vi "simple-LevyLab Analysis Framework (Template).vi"() -> ()   [LabVIEW 2016]
doc: "simple-LevyLab Analysis Framework (s-LLAF).\n\nDrag onto an empty block diagram to make your own."
uses:
  <userlib>/LevyLab/XY Utilities/Typedefs/Interpolation Configuration--cluster.ctl
  <userlib>/LevyLab/Graph Utilities/graph_utilities.lvclass
  <userlib>/LevyLab/Graph Utilities/graph_utilities.lvclass/graph_utilities.ctl
  <userlib>/LevyLab/Graph Utilities/XY Graph/Set XY Graph Value (array).vi
  <userlib>/LevyLab/XY Utilities/subVIs/Add float (multiple).vi
  <userlib>/LevyLab/XY Utilities/subVIs/Subtract float (multiple).vi
  <userlib>/LevyLab/XY Utilities/subVIs/Multiply float (multiple).vi
  <userlib>/LevyLab/XY Utilities/subVIs/Square (multiple).vi
  <userlib>/LevyLab/XY Utilities/subVIs/Divide float (multiple).vi
  <userlib>/LevyLab/XY Utilities/subVIs/Sort (multiple).vi
  <userlib>/LevyLab/XY Utilities/subVIs/Swap X and Y (multiple).vi
  <userlib>/LevyLab/XY Utilities/subVIs/Reverse (multiple).vi
  <userlib>/LevyLab/XY Utilities/subVIs/Subset (multiple).vi
  <userlib>/LevyLab/XY Utilities/subVIs/Derivative (multiple).vi
  <userlib>/LevyLab/XY Utilities/subVIs/Interpolate (multiple).vi
  <userlib>/LevyLab/XY Utilities/subVIs/FFT (multiple).vi
  <userlib>/LevyLab/XY Utilities/subVIs/PS (multiple).vi
  <userlib>/LevyLab/XY Utilities/subVIs/Resample (multiple).vi
  <userlib>/LevyLab/XY Utilities/subVIs/Symmetrize (multiple).vi
  <userlib>/LevyLab/XY Utilities/xy_utilities.lvlib
panel:
  in  "Tab Control":enum32{"Page 1", "Page 2"}(tab)
  in  "STOP":bool
  in  "CLEAR":bool
  out "Current State":string="XY: Load\nGraph: Initialize Graphs\nUI: Display Data"
  in  "Method":enum16{"Slider (%)", "X[] min and max"}(ring)
  in  "Subset Slider":cluster{dbl, dbl}(slide)={0.75, 0.25} caption="Horizontal Slider" scale=0.0..1.0
  in  "Interval":dbl=2.0
  in  "Type":enum16{"dy/dx vs x", "dx/dy vs y"}(ring)
  in  "PROCESS":bool
  in  "Process Queue":string
  in  "Available States":i32(listbox)=-1 caption="States to Process"
  in  "x":dbl format="%#_6p"
  in  "y":dbl format="%#_6p"
  out "Processed States":string="XY: Load\nGraph: Initialize Graphs\nUI: Display Data"
  in  "Interval Units":enum16{"Points", "Data"}(ring)
  in  "Configure":T1={"X Low"=0.05, "X High"=0.5, "X Step"=0.01, "Fake Point"=0.05} {"Fake Point" format="%#_6p"; "X Step" format="%#_6p"; "X High" format="%#_6p"; "X Low" format="%#_6p"}
  in  "Graphs Tab Control":enum32{"Data", "Intensity/Linecuts"}(tab)
  out "XY Graph: Antisymmetric":cluster{"X-array":dbl[], dbl[]}[](graph)
  out "XY Graph: Symmetric":cluster{"X-array":dbl[], dbl[]}[](graph)
  out "XY Graph: Processed":cluster{"Intensity Data":dbl[], "Array":dbl[]}[](graph)
  out "XY Graph: Unprocessed":cluster{"Intensity Data":dbl[], "Array":dbl[]}[](graph)
  out "Data Intensity":dbl[][](graph)
  out "Diff Intensity":dbl[][](graph)
  out "Diff Vertical":cluster{"Array":dbl[], "A x Vector":dbl[]}[](graph)
  out "Diff Horizontal":cluster{"Array":dbl[], "A x Vector":dbl[]}[](graph)
  in  "width (vertical)":dbl=0.2 caption="width"
  in  "width (horizontal)":dbl=0.2 caption="width"
  in  "width (vertical) 2":dbl=0.2 caption="width"
  in  "width (horizontal) 2":dbl=0.2 caption="width"
  out "Data Vertical":cluster{"Array":dbl[], "A x Vector":dbl[]}[](graph)
  out "Data Horizontal":cluster{"Intensity Data":dbl[], "Array":dbl[]}[](graph)
  # "State Scripting"
  # "Process Arguments"
  # "Arithmetic"
  # "Derivative"
  # "Interpolate"
  # "Subset"
  # "\"Process Queue\" is a list of states that will execute when you press the \"PROCESS\" button. (File: Load and Graph: Update Graph are added automatically to the beginning and end of the queue.)\n\nTo add states you can either:\n- Type directly into the Process Queue box.\nor:\n- Select a state in the \"Available States\" box that you want to add to the queue. ctl-v in the \"Process Queue\" control to add to the queue."
  # "XY Graphs"
  # "Symmeterized Graphs"
  # "Data processing (1)"
  # "Data Processing (2)"
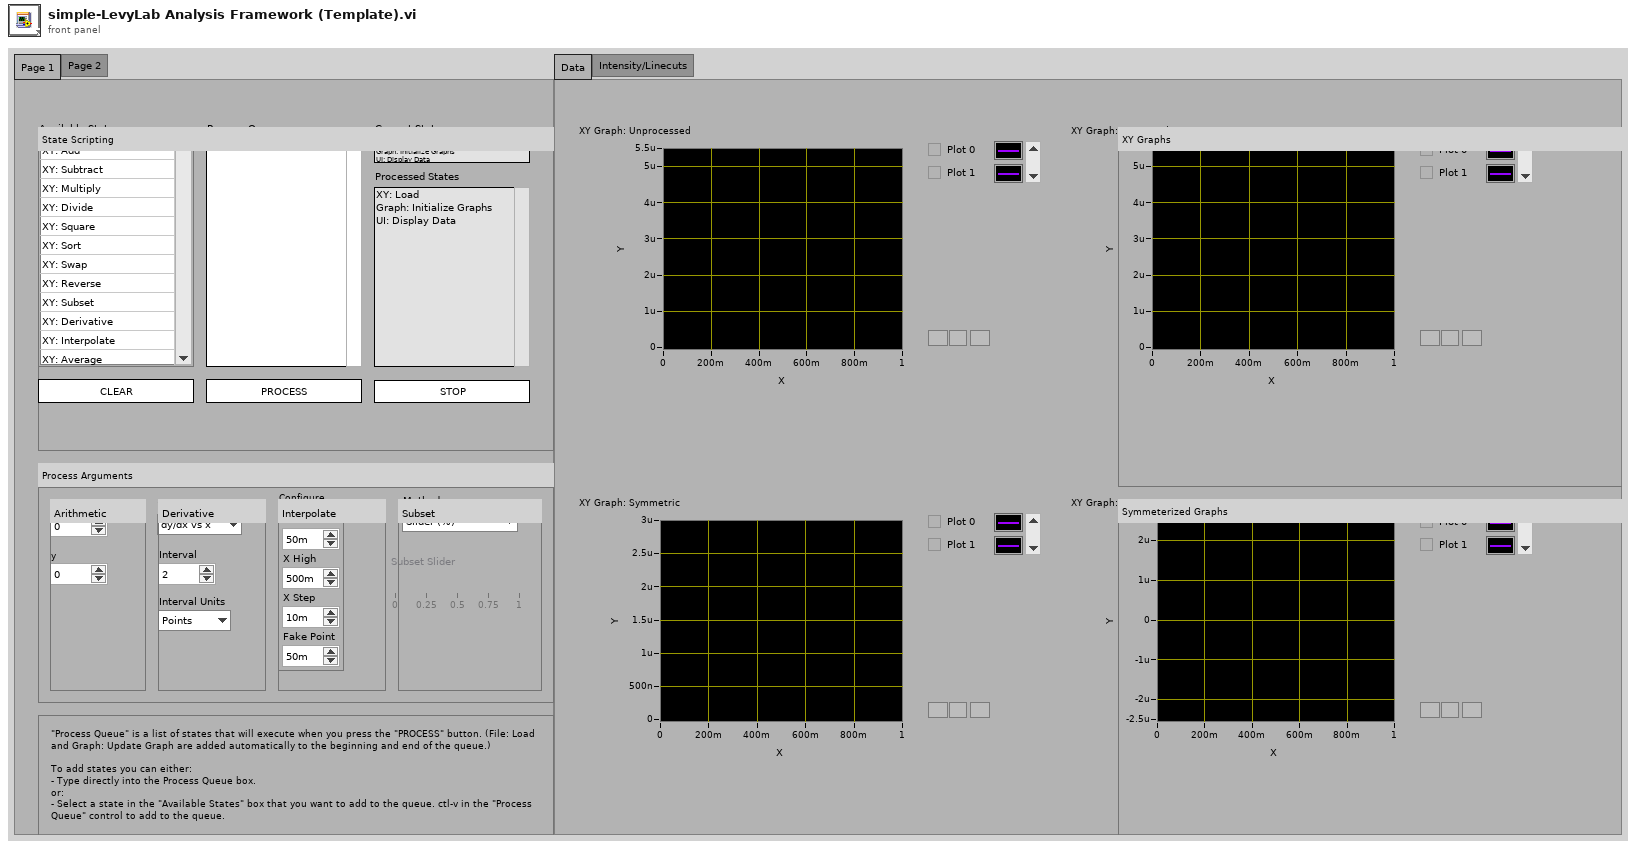
[diagram p1: front panel]
types:
  T1 = typedef "xy_utilities.lvlib/Interpolation Configuration--cluster.ctl" = cluster{"X Low":dbl, "X High":dbl, "X Step":dbl, "Fake Point":dbl}
  T2 = enum32{"Invalid", "Standard", "Closed", "Hidden", "Minimized", "Maximized"}
  T3 = enum32{"invalid app kind", "Development System", "Run Time System", "Student Edition", "Embedded LabVIEW", "Evaluation", "Custom"}
  T4 = cluster{"Shift":bool, "Ctrl":bool, "Alt":bool, "Cmd":bool, "Opt":bool}
  T5 = cluster{"Core":cluster{"Current VI Reference":refnum<vi>, "Close Panel on Exit?":bool}, "Graph":cluster{"Data: Unprocessed":refnum<class "graph_utilities.lvclass">, "Data: Processed":refnum<class "graph_utilities.lvclass">, "Data: Intensity/Vertical":refnum<class "graph_utilities.lvclass">, "Data: Intensity/Horizontal":refnum<class "graph_utilities.lvclass">, "Differential: Intensity/Vertical":refnum<class "graph_utilities.lvclass">, "Differential: Intensity/Horizontal":refnum<class "graph_utilities.lvclass">}, "XY Data (unprocessed)":cluster{"Intensity Data":dbl[], "Array":dbl[]}[], "XY Data (processed 1)":cluster{"Intensity Data":dbl[], "Array":dbl[]}[], "XY Data (processed 2)":cluster{"Intensity Data":dbl[], "Array":dbl[]}[], "Parameter":dbl[]}
  T6 = cluster{"Data: Unprocessed":refnum<class "graph_utilities.lvclass">, "Data: Processed":refnum<class "graph_utilities.lvclass">, "Data: Intensity/Vertical":refnum<class "graph_utilities.lvclass">, "Data: Intensity/Horizontal":refnum<class "graph_utilities.lvclass">, "Differential: Intensity/Vertical":refnum<class "graph_utilities.lvclass">, "Differential: Intensity/Horizontal":refnum<class "graph_utilities.lvclass">}
  T7 = cluster{"Current VI Reference":refnum<vi>, "Close Panel on Exit?":bool}
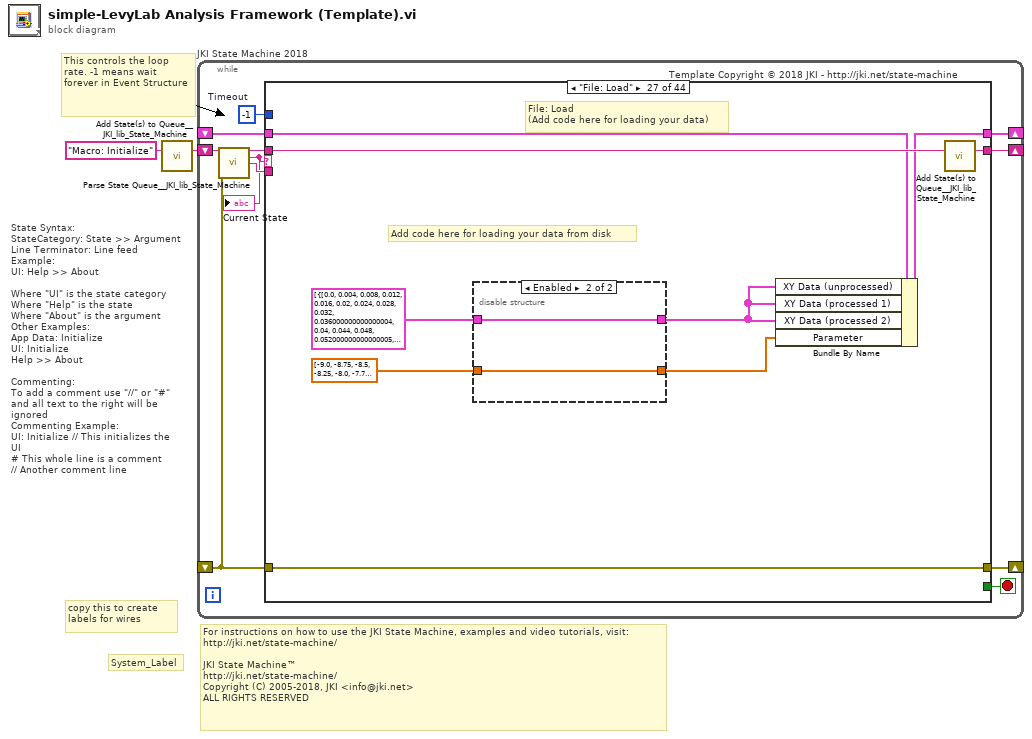
[diagram p0: block diagram]
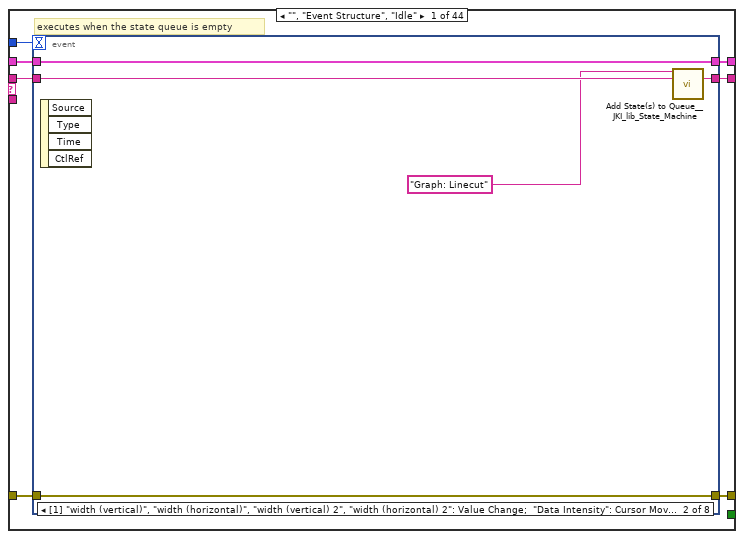
[diagram p2: hidden frame]
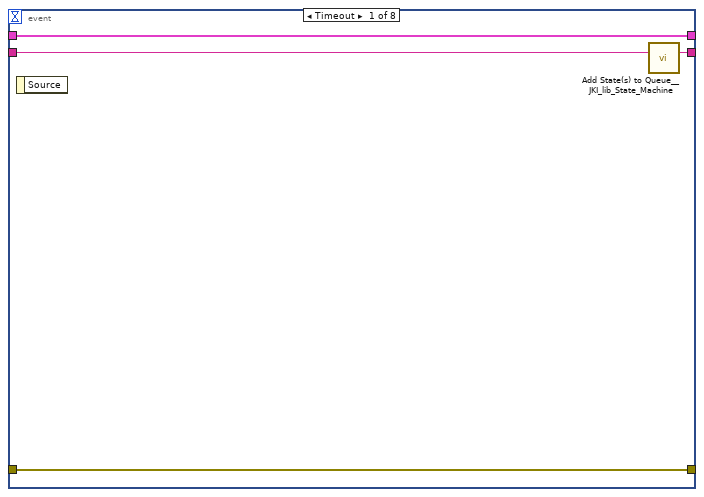
[diagram p3: hidden frame]
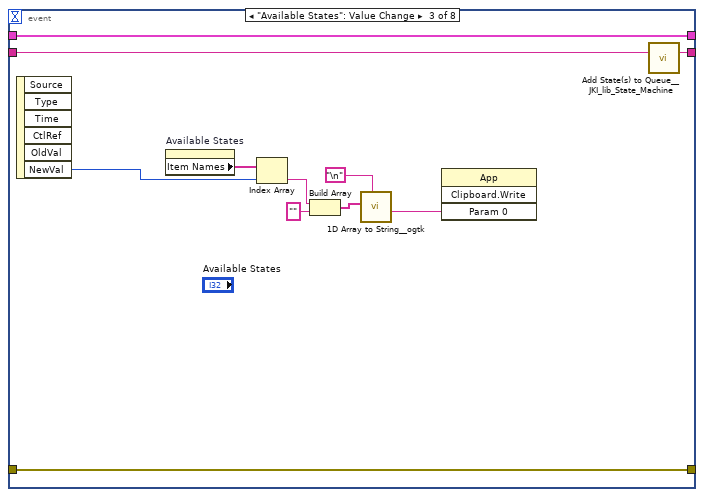
[diagram p4: hidden frame]
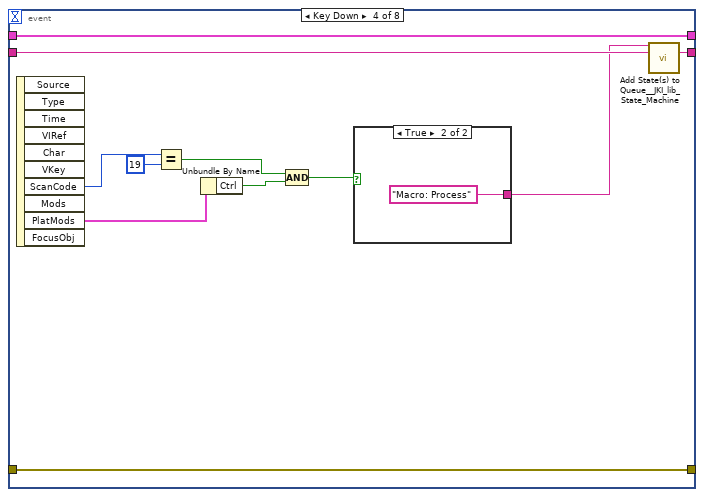
[diagram p5: hidden frame]
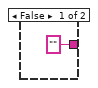
[diagram p6: hidden frame]
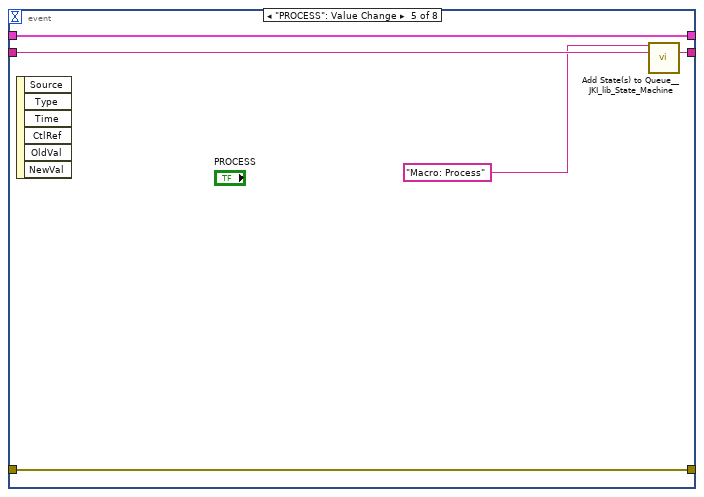
[diagram p7: hidden frame]
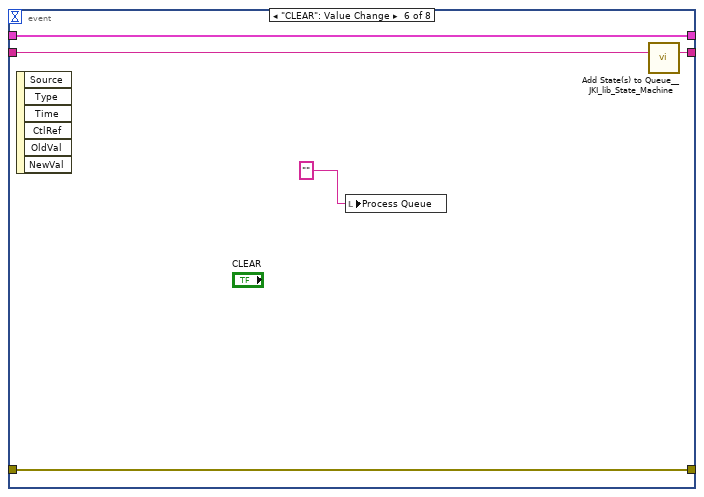
[diagram p8: hidden frame]
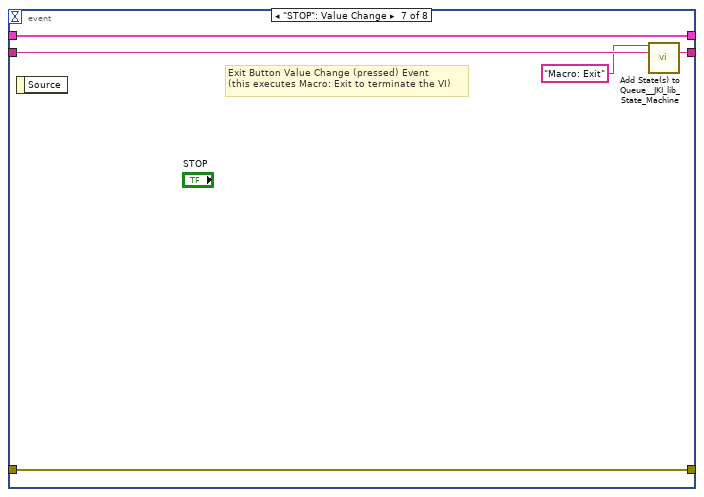
[diagram p9: hidden frame]
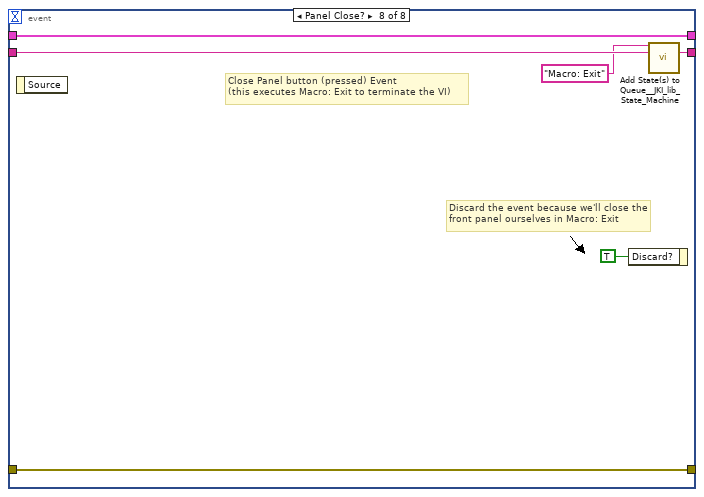
[diagram p10: hidden frame]
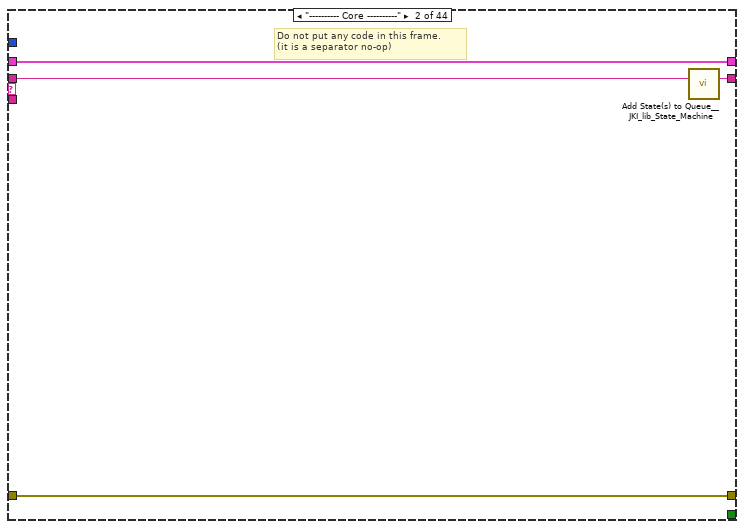
[diagram p11: hidden frame]
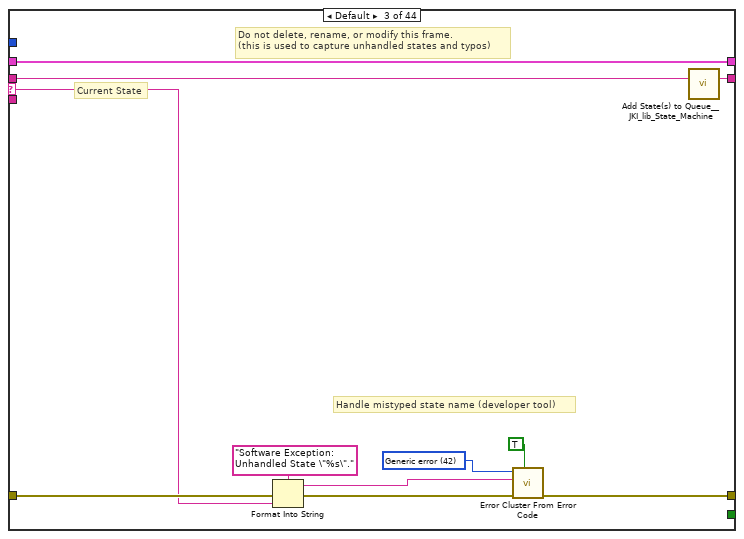
[diagram p12: hidden frame]
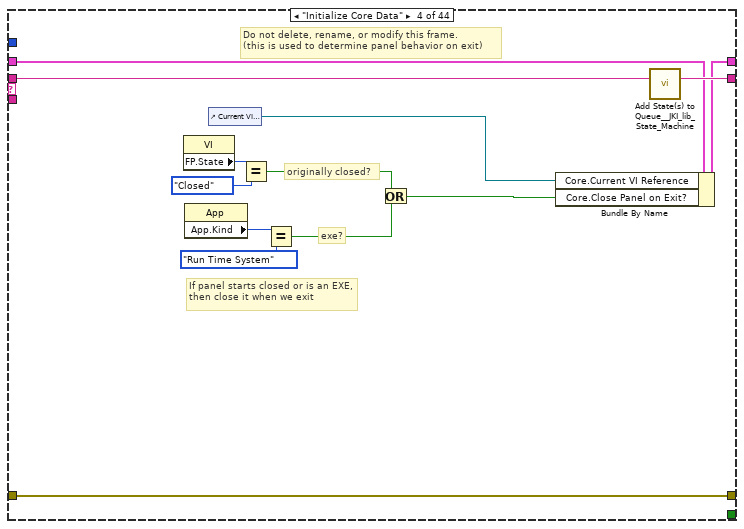
[diagram p13: hidden frame]
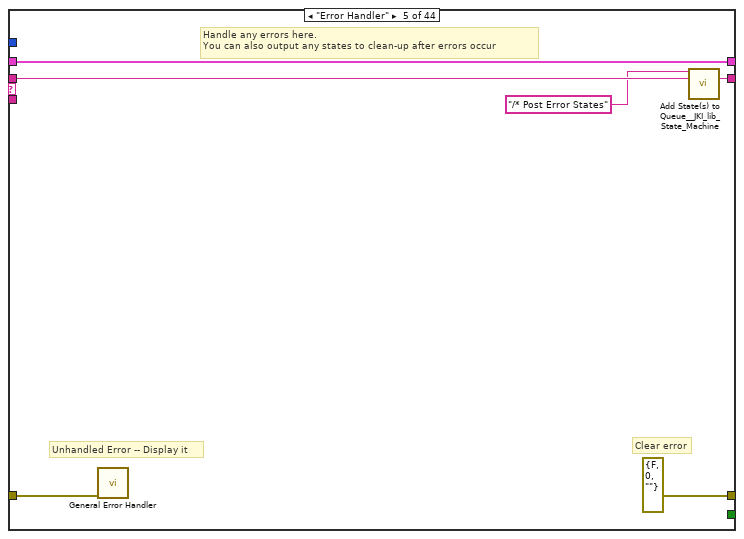
[diagram p14: hidden frame]
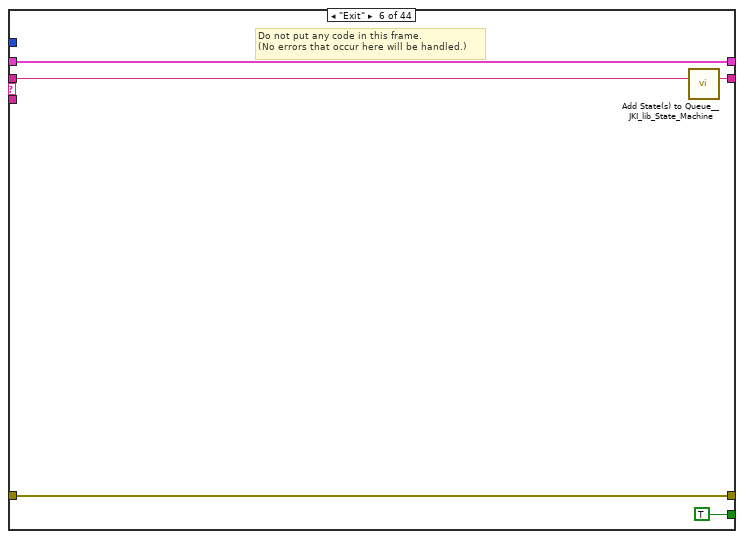
[diagram p15: hidden frame]
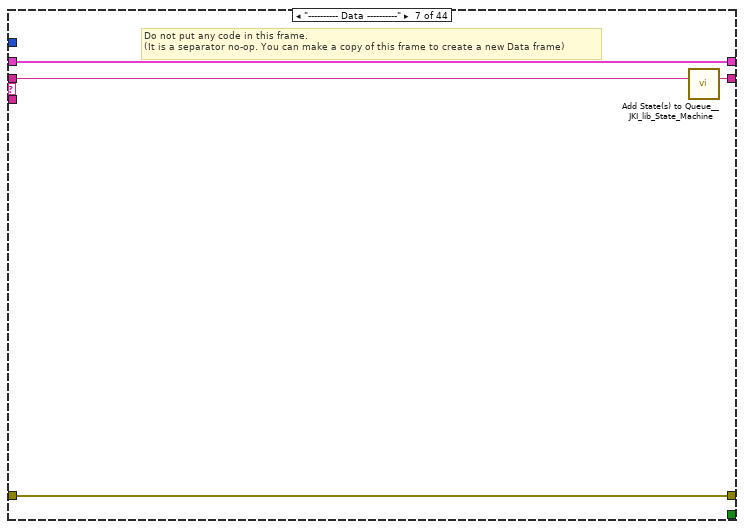
[diagram p16: hidden frame]
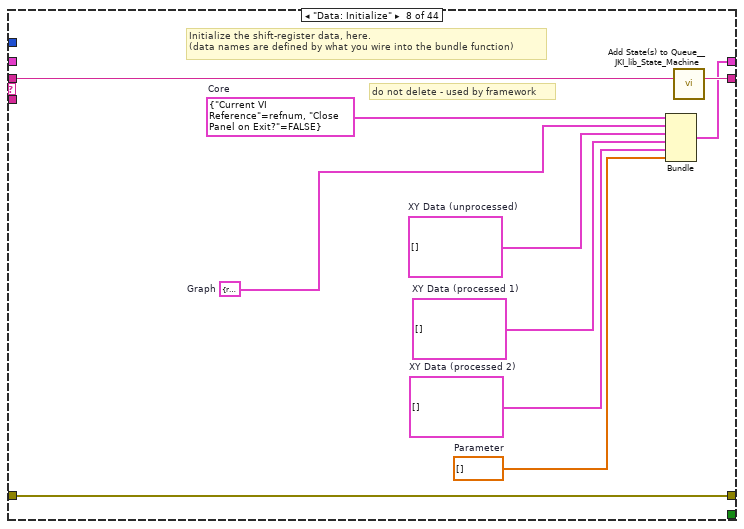
[diagram p17: hidden frame]
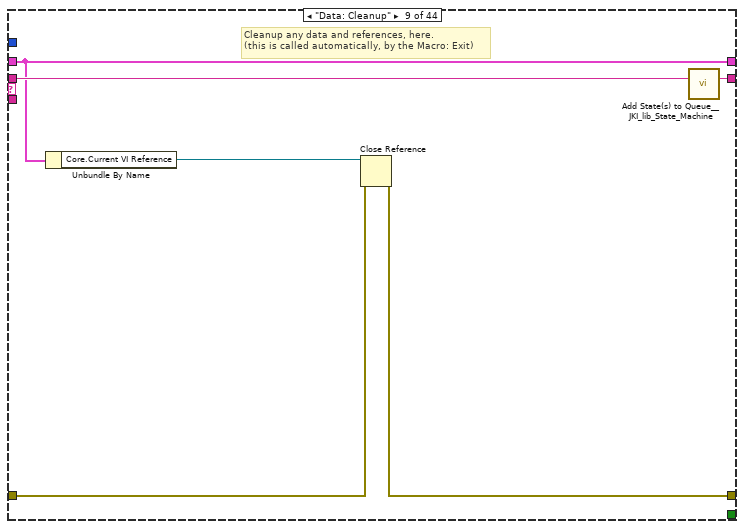
[diagram p18: hidden frame]
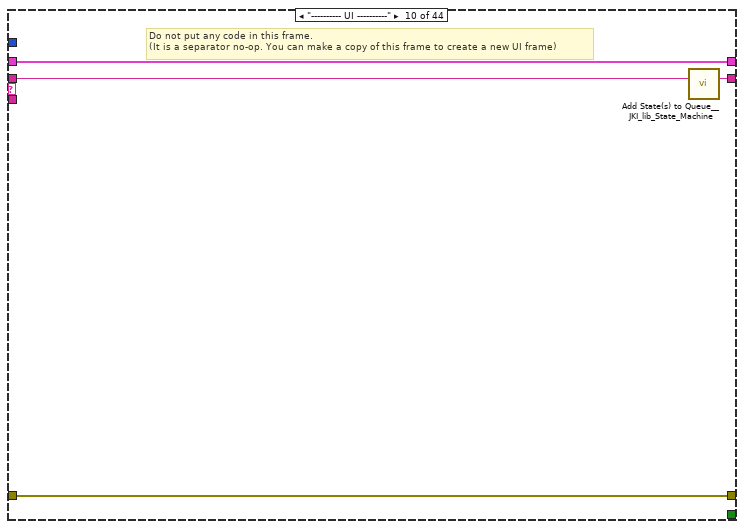
[diagram p19: hidden frame]
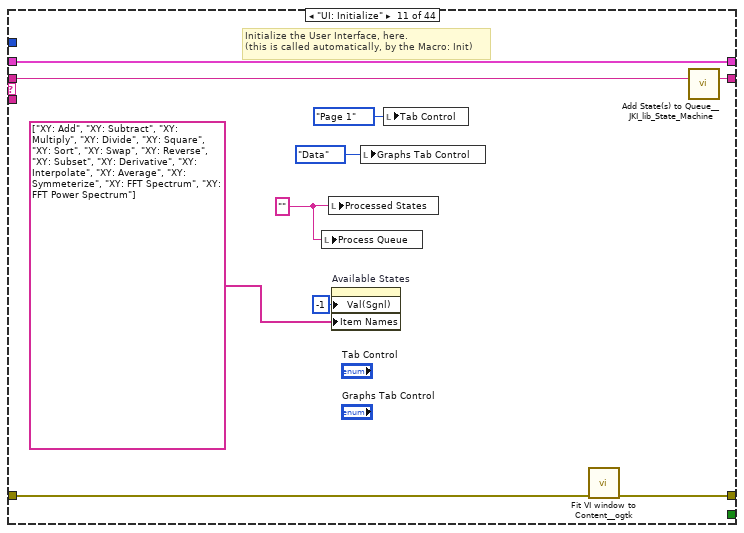
[diagram p20: hidden frame]
diagram:
  # "For instructions on how to use the JKI State Machine, examples and video tutorials, visit:\nhttp://jki.net/state-machine/\n\nJKI State Machine™\nhttp://jki.net/state-machine/\nCopyright (C) 2005-2018, JKI <info@jki.net>\nALL RIGHTS RESERVED"
  # "State Syntax:\nStateCategory: State >> Argument\nLine Terminator: Line feed\nExample:\nUI: Help >> About\n\nWhere \"UI\" is the state category\nWhere \"Help\" is the state\nWhere \"About\" is the argument\nOther Examples:\nApp Data: Initialize\nUI: Initialize\nHelp >> About\n\nCommenting:\nTo add a comment use \"//\" or \"#\" and all text to the right will be ignored\nCommenting Example:\nUI: Initialize // This initializes the UI\n# This whole line is a comment\n// Another comment line"
  # "copy this to create labels for wires"
  # "This controls the loop rate. -1 means wait forever in Event Structure"
  # "System_Label"
  n1 = call <vilib>:"Add State(s) to Queue__JKI_lib_State_Machine.vi"("State(s) in (\"\")"="Macro: Initialize") -> ("States Out"=w2:string)  [unwired: 14 in]
  n2 = while "JKI State Machine 2018" {
    shift-right: [w7] -> _
    shift-left: _ -> [w6]
    shift-right: [w10] -> _
    shift-left: _ -> [w4]
    shift-right: [w9] -> _
    shift-left: w2 -> [w11]
    stop <- w8 stop-if-true
    w5 = -1  # Timeout
    # "Template Copyright © 2018 JKI - http://jki.net/state-machine"
    n3 = call <vilib>:"Parse State Queue__JKI_lib_State_Machine.vi"("State Queue"=w11, "Error In (no error)"=w4) -> ("Remaining States"=w13:string, "Current State"=w3:string, "Arguments"=w12:string)  [unwired: 11 in]
    "Current State" <- w3
    n4 = case shown="\"File: Load\"" w3 {
      selector: w3 -> [_ _ w79 _ _ _ _ _ _ _ _ _ _ _ _ _ _ _ _ _ _ _ _ _ _ _ _ _ _ _ _ _ _ _ _ _ _ _ _ _ _ _ _ _]
      tunnel: w13 -> [w20 w78 w83 w102 w108 w113 w117 w127 w133 w137 w147 w153 w164 w233 w238 w248 w256 w260 w264 w281 w305 w315 w325 w349 w365 w369 w378 w392 w402 w412 w422 w430 w440 w448 w456 w464 w474 w485 w494 w502 w510 w518 w526 w536]
      tunnel: w12 -> [_ _ _ _ _ _ _ _ _ _ _ w148 w158 _ _ _ _ _ _ _ _ _ _ _ _ _ _ _ _ _ _ _ _ _ _ _ _ _ _ _ _ _ _ _]
      tunnel: w6 -> [w18 w75 w81 w95 w105 w111 w114 _ w128 w134 w145 w151 w160 w230 w235 w245 w253 w257 w261 w279 w303 w310 w323 w346 w363 w366 w373 w389 w399 w409 w419 w427 w437 w445 w453 w461 w471 w482 w491 w499 w507 w515 w523 w533]
      tunnel: [w17 w76 w85 w99 errorcluster {"status"=FALSE, "code"=0, "source"=""} ("error out") w110 w115 w124 w129 w135 w138 w149 w161 w231 w236 w246 w254 w258 w262 w277 w288 w306 w316 w347 w354 w367 w370 w385 w395 w405 w415 w423 w433 w441 w449 w457 w467 w479 w487 w495 w504 w511 w519 w529] -> w10
      tunnel: w4 -> [w16 w76 w84 w99 w104 w110 w115 w124 w130 w135 w139 w150 w162 w231 w236 w246 w254 w258 w262 w268 w282 w309 w320 w347 w356 w367 w370 w386 w396 w406 w416 w424 w434 w442 w450 w458 w468 w480 w488 w496 w505 w512 w520 w530]
      tunnel: [w19 w77 w82 w101 w107 w112 w116 w126 w132 w136 w146 w152 w163 w232 w237 w247 w255 w259 w263 w280 w304 w314 w324 w348 w364 w368 w377 w391 w401 w411 w421 w429 w439 w447 w455 w463 w473 w484 w493 w501 w509 w517 w525 w535] -> w9
      tunnel: [_ _ _ _ _ TRUE _ _ _ _ _ _ _ _ _ _ _ _ _ _ _ _ _ _ _ _ _ _ _ _ _ _ _ _ _ _ _ _ _ _ _ _ _ _] -> w8
      tunnel: [w15 w75 w81 w100 w105 w111 w114 w125 w128 w134 w145 w151 w160 w230 w235 w245 w253 w257 w261 w278 w302 w310 w323 w346 w363 w366 w376 w388 w398 w408 w418 w426 w436 w444 w452 w460 w470 w481 w490 w498 w506 w514 w522 w532] -> w7
      tunnel: w5 -> [w14 _ _ _ _ _ _ _ _ _ _ _ _ _ _ _ _ _ _ _ _ _ _ _ _ _ _ _ _ _ _ _ _ _ _ _ _ _ _ _ _ _ _ _]
      frame "", "Event Structure", "Idle" {
        # "executes when the state queue is empty"
        n5 = event shown="[1] \"width (vertical)\", \"width (horizontal)\", \"width (vertical) 2\", \"width (horizontal) 2\": Value Change;  \"Data Intensity\": Cursor Move" {
          selector: _ -> [_ _ _ _ _ _ _ _]
          dyn-events: _ -> [_ _ _ _ _ _ _ _]
          timeout: w14 -> [_ _ _ _ _ _ _ _]
          tunnel: w20 -> [w24 w29 w40 w51 w58 w63 w68 w74]
          tunnel: [w23 w28 w39 w50 w57 w62 w67 w73] -> w19
          tunnel: w18 -> [w21 w26 w37 w48 w55 w60 w65 w71]
          tunnel: [w22 w27 w38 w49 w56 w61 w66 w72] -> w17
          tunnel: w16 -> [w22 w27 w38 w49 w56 w61 w66 w72]
          tunnel: [w21 w26 w37 w48 w55 w60 w65 w71] -> w15
          event Timeout {
            n6 = event-data() -> ()  [unwired: 1 in, 1 out]
            n7 = call <vilib>:"Add State(s) to Queue__JKI_lib_State_Machine.vi"("State(s) in (\"\")"=w24) -> ("States Out"=w23:string)  [unwired: 14 in]
          }
          event "width (vertical)", "width (horizontal)", "width (vertical) 2", "width (horizontal) 2": Value Change; "Data Intensity": Cursor Move {
            n8 = event-data() -> ()  [unwired: 1 in, 4 out]
            n9 = call <vilib>:"Add State(s) to Queue__JKI_lib_State_Machine.vi"("State(s) in Front (\"\")"="Graph: Linecut" ("State(s) in Front (\"\")"), "State(s) in (\"\")"=w29) -> ("States Out"=w28:string)  [unwired: 13 in]
          }
          event "Available States": Value Change {
            n10 = event-data() -> ("NewVal"=w31:i32)  [unwired: 1 in, 5 out]
            n11 = property on="Available States" class="LstBox (strict)"() -> ("Item Names"=w32:string[])  [unwired: 2 in, 2 out]
            n12 = Index Array(array=w32, index=w31) -> (element=w36:string)
            n13 = Build Array(w36, "" ("element")) -> (w33:string[])
            n14 = call <userlib>:"1D Array to String__ogtk.vi"("delimiter (Tab)"="\n", "Array of Strings"=w33) -> ("delimited string"=w34:string)  [unwired: 9 in]
            n15 = invoke class="App" method="Clipboard.Write"("Param 0"=w34) -> ()  [unwired: 3 in, 4 out]
            n16 = call <vilib>:"Add State(s) to Queue__JKI_lib_State_Machine.vi"("State(s) in (\"\")"=w40) -> ("States Out"=w39:string)  [unwired: 14 in]
          }
          event Key Down {
            n17 = event-data() -> ("ScanCode"=w41:i16, "PlatMods"=w42:T4)  [unwired: 1 in, 8 out]
            n18 = Equal?(x=w41, y=i16 19) -> (x = y?=w44:bool)
            n19 = Unbundle By Name(w42) -> ("Ctrl"=w45:bool)
            n20 = Compound Arithmetic op=AND(w44, w45) -> (w43:bool)
            n21 = case shown="True" w43 {
              tunnel: ["" ("State(s) in Front (\"\")") "Macro: Process" ("State(s) in Front (\"\")")] -> w46
              frame False {
              }
              frame True {
              }
            }
            n22 = call <vilib>:"Add State(s) to Queue__JKI_lib_State_Machine.vi"("State(s) in Front (\"\")"=w46, "State(s) in (\"\")"=w51) -> ("States Out"=w50:string)  [unwired: 13 in]
          }
          event "PROCESS": Value Change {
            n23 = event-data() -> ()  [unwired: 1 in, 6 out]
            n24 = call <vilib>:"Add State(s) to Queue__JKI_lib_State_Machine.vi"("State(s) in Front (\"\")"="Macro: Process" ("State(s) in Front (\"\")"), "State(s) in (\"\")"=w58) -> ("States Out"=w57:string)  [unwired: 13 in]
          }
          event "CLEAR": Value Change {
            n25 = event-data() -> ()  [unwired: 1 in, 6 out]
            n26 = local write "Process Queue"("" ("Process States")) -> ()
            n27 = call <vilib>:"Add State(s) to Queue__JKI_lib_State_Machine.vi"("State(s) in (\"\")"=w63) -> ("States Out"=w62:string)  [unwired: 14 in]
          }
          event "STOP": Value Change {
            # "Exit Button Value Change (pressed) Event\n(this executes Macro: Exit to terminate the VI)"
            n28 = event-data() -> ()  [unwired: 1 in, 1 out]
            n29 = call <vilib>:"Add State(s) to Queue__JKI_lib_State_Machine.vi"("State(s) in Front (\"\")"="Macro: Exit", "State(s) in (\"\")"=w68) -> ("States Out"=w67:string)  [unwired: 13 in]
          }
          event Panel Close? {
            # "Discard the event because we'll close the front panel ourselves in Macro: Exit"
            # "Close Panel button (pressed) Event\n(this executes Macro: Exit to terminate the VI)"
            n30 = event-data() -> ()  [unwired: 1 in, 1 out]
            n31 = event-data("Discard?"=TRUE) -> ()  [unwired: 1 in, 1 out]
            n32 = call <vilib>:"Add State(s) to Queue__JKI_lib_State_Machine.vi"("State(s) in Front (\"\")"="Macro: Exit", "State(s) in (\"\")"=w74) -> ("States Out"=w73:string)  [unwired: 13 in]
          }
        }
      }
      frame "---------- Core ----------" {
        # "Do not put any code in this frame.\n(it is a separator no-op)"
        n33 = call <vilib>:"Add State(s) to Queue__JKI_lib_State_Machine.vi"("State(s) in (\"\")"=w78) -> ("States Out"=w77:string)  [unwired: 14 in]
      }
      frame Default {
        w88 = 42 items=["No error", "Argument error", "Memory is full", "Out of zone", "End of file", "File already open", "Generic file I/O error", "File not found", "File permission error", "Disk is full", "Duplicate path", "Too many files open", "System feature not enabled", "Resource file not found", "Cannot add resource", "Resource not found", "Image not found", "Image memory error", "Pen does not exist", "Config type invalid", "Config token not found", "Config parse error", "Config memory error", "Bad external code format", "Bad external code offset", "External code not present", "Null window", "Destroy window error", "Null menu", "Print aborted", "Bad print record", "Print driver error", "Windows error during printing", "Memory error during printing", "Print dialog error", "Generic print error", "Invalid device refnum", "Device not found", "Device parameter error", "Device unit error", "Cannot open device", "Device call aborted", "Generic error", "Cancelled by user", "Object ID too low", "Object ID too high", "Object not in heap", "Unknown heap", "Unknown object (invalid DefProc)", "Unknown object (DefProc not in table)", "Message out of range", "Invalid (null) method", "Unknown message", "Manager call not supported", "Bad address", "Network operation in progress", "Network operation timed out", "Connection is busy", "Network attribute not supported", "Network error", "Address in use", "System out of memory", "Connection aborted", "Connection refused", "Not connected", "Already connected", "Connection closed", "Initialization error (interapplication manager)", "Bad occurrence", "Wait on unbound occurrence handler", "Occurrence queue overflow", "Datalog type conflict", "Unused", "Unrecognized type (interapplication manager)", "Memory corrupt", "Failed to make temporary DLL", "Old CIN version", "Drag socket not found", "Failed to load drop-object", "Failed to register OLE object", "Failed to release OLE object", "Format specifier type mismatch", "Unknown format specifier", "Too few format specifiers", "Too many format specifiers", "Scan failed", "Newer CIN version", "Error converting to variant", "Runtime menu error", "Password tampered", "Variant attribute not found", "Incompatible variant data type", "Event data is not available", "Event Store is not present", "Occurrence is not found", "Event Queue is not created", "Event info is not available", "Refnum passed is NULL", "Error retrieving Class GUID", "Error retrieving CoClass GUID", "Error retrieving TypeLib GUID.", "Bad built application magic bytes.", "Specific driver is different from the specific driver associated with the Logical Name.", "There is no session opened to the class driver.", "Max Error", "MAX - Error with config objects", "MAX - Error loading configuration", "MAX - Group not supported"]
        # "Current State"
        # "Do not delete, rename, or modify this frame.\n(this is used to capture unhandled states and typos)"
        # "Handle mistyped state name (developer tool)"
        n34 = Format Into String(format string="Software Exception: Unhandled State \"%s\"." ("message"), error in=w84, w79) -> (resulting string=w87:string, error out=w86:errorcluster)  [unwired: 1 in]
        n35 = call <vilib>:"Error Cluster From Error Code.vi"("show call chain? (False)"=TRUE, "error in (no error)"=w86, "error message (\"\")"=w87, "error code (0)"=w88) -> ("error out"=w85:errorcluster)  [unwired: 5 in]
        n36 = call <vilib>:"Add State(s) to Queue__JKI_lib_State_Machine.vi"("State(s) in (\"\")"=w83) -> ("States Out"=w82:string)  [unwired: 14 in]
      }
      frame "Initialize Core Data" {
        # "Do not delete, rename, or modify this frame.\n(this is used to determine panel behavior on exit)"
        # "originally closed?"
        # "exe?"
        # "If panel starts closed or is an EXE, then close it when we exit"
        n37 = property class="VI"() -> ("FP.State"=w92:T2)  [unwired: 2 in, 2 out]
        n38 = property class="App"() -> ("App.Kind"=w98:T3)  [unwired: 2 in, 2 out]
        n39 = control-ref of="Current VI Reference"() -> (w93:refnum<vi>)
        n40 = Equal?(x=w92, y=T2."Closed" ("Front Panel Window:State")) -> (x = y?=w90:bool)
        n41 = Equal?(x=w98, y=T3."Run Time System" ("Application:Kind")) -> (x = y?=w96:bool)
        n42 = Or(x=w90, y=w96) -> (x .or. y?=w94:bool)
        n43 = Bundle By Name(cluster=w95, "Core.Current VI Reference"=w93, "Core.Close Panel on Exit?"=w94) -> (w100:T5)
        n44 = call <vilib>:"Add State(s) to Queue__JKI_lib_State_Machine.vi"("State(s) in (\"\")"=w102) -> ("States Out"=w101:string)  [unwired: 14 in]
      }
      frame "Error Handler" {
        # "Unhandled Error -- Display it"
        # "Handle any errors here.\nYou can also output any states to clean-up after errors occur"
        # "Clear error"
        n45 = call <vilib>:"General Error Handler.vi"("error in (no error)"=w104) -> ()  [unwired: 10 in, 5 out]
        n46 = call <vilib>:"Add State(s) to Queue__JKI_lib_State_Machine.vi"("State(s) in Front (\"\")"="/* Post Error States", "State(s) in (\"\")"=w108) -> ("States Out"=w107:string)  [unwired: 13 in]
      }
      frame "Exit" {
        # "Do not put any code in this frame.\n(No errors that occur here will be handled.)"
        n47 = call <vilib>:"Add State(s) to Queue__JKI_lib_State_Machine.vi"("State(s) in (\"\")"=w113) -> ("States Out"=w112:string)  [unwired: 14 in]
      }
      frame "---------- Data ----------" {
        # "Do not put any code in this frame.\n(It is a separator no-op. You can make a copy of this frame to create a new Data frame)"
        n48 = call <vilib>:"Add State(s) to Queue__JKI_lib_State_Machine.vi"("State(s) in (\"\")"=w117) -> ("States Out"=w116:string)  [unwired: 14 in]
      }
      frame "Data: Initialize" {
        w118 = T6 {"Data: Unprocessed"=refnum, "Data: Processed"=refnum, "Data: Intensity/Vertical"=refnum, "Data: Intensity/Horizontal"=refnum, "Differential: Intensity/Vertical"=refnum, "Differential: Intensity/Horizontal"=refnum}  # Graph
        w119 = cluster{"Intensity Data":dbl[], "Array":dbl[]}[] []  # XY Data (processed 2)
        w120 = dbl[] []  # Parameter
        w121 = cluster{"Intensity Data":dbl[], "Array":dbl[]}[] []  # XY Data (processed 1)
        w122 = cluster{"Intensity Data":dbl[], "Array":dbl[]}[] []  # XY Data (unprocessed)
        w123 = T7 {"Current VI Reference"=refnum, "Close Panel on Exit?"=FALSE}  # Core
        # "do not delete - used by framework"
        # "Initialize the shift-register data, here.\n(data names are defined by what you wire into the bundle function)"
        n49 = Bundle("Core"=w123, "Graph"=w118, "XY Data (unprocessed)"=w122, "XY Data (processed 1)"=w121, "XY Data (processed 2)"=w119, "Parameter"=w120) -> (w125:T5)  [unwired: 1 in]
        n50 = call <vilib>:"Add State(s) to Queue__JKI_lib_State_Machine.vi"("State(s) in (\"\")"=w127) -> ("States Out"=w126:string)  [unwired: 14 in]
      }
      frame "Data: Cleanup" {
        # "Cleanup any data and references, here.\n(this is called automatically, by the Macro: Exit)"
        n51 = Unbundle By Name(w128) -> ("Core.Current VI Reference"=w131:refnum<vi>)
        n52 = Close Reference(reference=w131, error in (no error)=w130) -> (error out=w129:errorcluster)
        n53 = call <vilib>:"Add State(s) to Queue__JKI_lib_State_Machine.vi"("State(s) in (\"\")"=w133) -> ("States Out"=w132:string)  [unwired: 14 in]
      }
      frame "---------- UI ----------" {
        # "Do not put any code in this frame.\n(It is a separator no-op. You can make a copy of this frame to create a new UI frame)"
        n54 = call <vilib>:"Add State(s) to Queue__JKI_lib_State_Machine.vi"("State(s) in (\"\")"=w137) -> ("States Out"=w136:string)  [unwired: 14 in]
      }
      frame "UI: Initialize" {
        w141 = "" ("Process States")
        # "Initialize the User Interface, here.\n(this is called automatically, by the Macro: Init)"
        n55 = local write "Process Queue"(w141) -> ()
        n56 = local write "Processed States"(w141) -> ()
        n57 = property on="Available States" class="LstBox (strict)"("Val(Sgnl)"=-1 ("Value (Signaling)"), "Item Names"=string[] ["XY: Add", "XY: Subtract", "XY: Multiply", "XY: Divide", "XY: Square", "XY: Sort", "XY: Swap", "XY: Reverse", "XY: Subset", "XY: Derivative", "XY: Interpolate", "XY: Average", "XY: Symmeterize", "XY: FFT Spectrum", "XY: FFT Power Spectrum"]) -> ()  [unwired: 2 in, 2 out]
        n58 = local write "Graphs Tab Control"(enum32{"Data", "Intensity/Linecuts"}."Data" ("Graphs Tab Control")) -> ()
        n59 = local write "Tab Control"(enum32{"Page 1", "Page 2"}."Page 1" ("Tab Control")) -> ()
        n60 = call <userlib>:"Fit VI window to Content__ogtk.vi"("error in (no error)"=w139) -> ("error out"=w138:errorcluster)  [unwired: 5 in, 1 out]
        n61 = call <vilib>:"Add State(s) to Queue__JKI_lib_State_Machine.vi"("State(s) in (\"\")"=w147) -> ("States Out"=w146:string)  [unwired: 14 in]
      }
      frame "UI: Cursor Set" {
        # "Argument"
        # "Set and Unset Cursor Busy.\n(Usage: \"UI: Cursor Set >> Busy|Idle\")"
        n62 = case shown="\"Idle\", Default" w148 {
          tunnel: w150 -> [w155 w157]
          tunnel: [w154 w156] -> w149
          frame "Idle", Default {
            n63 = call <vilib>:"Unset Busy.vi"("error in (no error)"=w155) -> ("error out"=w154:errorcluster)  [unwired: 10 in]
          }
          frame "Busy" {
            n64 = call <vilib>:"Set Busy.vi"("error in (no error)"=w157) -> ("error out"=w156:errorcluster)  [unwired: 9 in, 1 out]
          }
        }
        n65 = call <vilib>:"Add State(s) to Queue__JKI_lib_State_Machine.vi"("State(s) in (\"\")"=w153) -> ("States Out"=w152:string)  [unwired: 14 in]
      }
      frame "UI: Front Panel State" {
        # "Argument"
        # "Set Front Panel Open or Closed\n(Usage: \"UI: Front Panel State >> Open|Close\")"
        n66 = Unbundle By Name(w160) -> ("Core.Current VI Reference"=w159:refnum<vi>)
        n67 = case shown="\"Maximize\", \"Maximized\"" w158 {
          tunnel: w162 -> [w170 w185 w196 w209 w222]
          tunnel: [w172 w186 w198 w211 w224] -> w161
          tunnel: w159 -> [w171 w183 w197 w210 w223]
          frame "Open", "Standard", Default {
            w165 = T2."Standard" ("State")
            n68 = property class="VI"(reference=w171, error in=w170) -> (reference out=w168:refnum<vi>, error out=w169:errorcluster, "FP.State"=w167:T2)
            n69 = Not Equal?(x=w167, y=w165) -> (x != y?=w166:bool)
            n70 = case shown="True" w166 {
              tunnel: [w176 w178] -> w172
              tunnel: w169 -> [w175 w178]
              tunnel: w168 -> [w174 _]
              tunnel: w165 -> [w173 _]
              frame True {
                n71 = invoke class="VI" method="FP.Open"(reference=w174, error in=w175, "Activate"=TRUE, "State"=w173) -> (error out=w176:errorcluster)  [unwired: 1 in, 4 out]
              }
              frame False {
              }
            }
          }
          frame "Close", "Closed" {
            n72 = property class="VI"(reference=w183, error in=w185) -> (reference out=w182:refnum<vi>, error out=w184:errorcluster, "FP.State"=w180:T2)
            n73 = Not Equal?(x=w180, y=T2."Closed" ("Front Panel Window:State")) -> (x != y?=w179:bool)
            n74 = case shown="True" w179 {
              tunnel: [w187 w190] -> w186
              tunnel: w184 -> [w187 w189]
              tunnel: w182 -> [_ w188]
              frame False {
              }
              frame True {
                n75 = invoke class="VI" method="FP.Close"(reference=w188, error in=w189) -> (error out=w190:errorcluster)  [unwired: 1 in, 2 out]
              }
            }
          }
          frame "Hidden", "Hide" {
            w191 = T2."Hidden" ("State")
            n76 = property class="VI"(reference=w197, error in=w196) -> (reference out=w194:refnum<vi>, error out=w195:errorcluster, "FP.State"=w193:T2)
            n77 = Not Equal?(x=w193, y=w191) -> (x != y?=w192:bool)
            n78 = case shown="True" w192 {
              tunnel: [w202 w203] -> w198
              tunnel: w195 -> [w201 w203]
              tunnel: w194 -> [w200 _]
              tunnel: w191 -> [w199 _]
              frame True {
                n79 = invoke class="VI" method="FP.Open"(reference=w200, error in=w201, "State"=w199) -> (error out=w202:errorcluster)  [unwired: 2 in, 4 out]
              }
              frame False {
              }
            }
          }
          frame "Minimize", "Minimized" {
            w204 = T2."Minimized" ("State")
            n80 = property class="VI"(reference=w210, error in=w209) -> (reference out=w207:refnum<vi>, error out=w208:errorcluster, "FP.State"=w206:T2)
            n81 = Not Equal?(x=w206, y=w204) -> (x != y?=w205:bool)
            n82 = case shown="True" w205 {
              tunnel: [w215 w216] -> w211
              tunnel: w208 -> [w214 w216]
              tunnel: w207 -> [w213 _]
              tunnel: w204 -> [w212 _]
              frame True {
                n83 = invoke class="VI" method="FP.Open"(reference=w213, error in=w214, "State"=w212) -> (error out=w215:errorcluster)  [unwired: 2 in, 4 out]
              }
              frame False {
              }
            }
          }
          frame "Maximize", "Maximized" {
            w217 = T2."Maximized" ("State")
            n84 = property class="VI"(reference=w223, error in=w222) -> (reference out=w220:refnum<vi>, error out=w221:errorcluster, "FP.State"=w219:T2)
            n85 = Not Equal?(x=w219, y=w217) -> (x != y?=w218:bool)
            n86 = case shown="True" w218 {
              tunnel: [w228 w229] -> w224
              tunnel: w221 -> [w227 w229]
              tunnel: w220 -> [w226 _]
              tunnel: w217 -> [w225 _]
              frame True {
                n87 = invoke class="VI" method="FP.Open"(reference=w226, error in=w227, "State"=w225) -> (error out=w228:errorcluster)  [unwired: 2 in, 4 out]
              }
              frame False {
              }
            }
          }
        }
        n88 = call <vilib>:"Add State(s) to Queue__JKI_lib_State_Machine.vi"("State(s) in (\"\")"=w164) -> ("States Out"=w163:string)  [unwired: 14 in]
      }
      frame "---------- Macro ----------" {
        # "Do not put any code in this frame.\n(It is a separator no-op. You can make a copy of this frame to create a new Macro frame)"
        n89 = call <vilib>:"Add State(s) to Queue__JKI_lib_State_Machine.vi"("State(s) in (\"\")"=w233) -> ("States Out"=w232:string)  [unwired: 14 in]
      }
      frame "Macro: Initialize" {
        # "Initialization Macro\n(This is called once, when the VI starts)"
        n90 = call <vilib>:"Add State(s) to Queue__JKI_lib_State_Machine.vi"("State(s) in Front (\"\")"="Data: Initialize\nInitialize Core Data\nUI: Initialize\nUI: Front Panel State >> Open\nGraph: Initialize References 1\nGraph: Initialize References 2", "State(s) in (\"\")"=w238) -> ("States Out"=w237:string)  [unwired: 13 in]
      }
      frame "Macro: Exit" {
        # "Exit Macro\n(This is called once, when the VI exits)"
        n91 = Unbundle By Name(w245) -> ("Core.Close Panel on Exit?"=w244:bool)
        n92 = Select(t="UI: Front Panel State >> Close", s=w244, f="") -> (s? t:f=w241:string)
        n93 = call <vilib>:"Add State(s) to Queue__JKI_lib_State_Machine.vi"("State(s) in (\"\")"=w241, "State(s) at Back (\"\")"="Graph: Clear\nData: Cleanup\nExit") -> ("States Out"=w239:string)  [unwired: 13 in]
        n94 = call <vilib>:"Add State(s) to Queue__JKI_lib_State_Machine.vi"("State(s) in Front (\"\")"=w239, "State(s) in (\"\")"=w248) -> ("States Out"=w247:string)  [unwired: 13 in]
      }
      frame "Macro: Process" {
        # "XY: Add\nXY: Subtract\nXY: Multiply\nXY: Divide\nXY: Sort\nXY: Swap\nXY: Reverse\nXY: Subset\nXY: Derivative\nXY: Interpolate\nXY: FFT Spectrum\nXY: FFT Power Spectrum"
        # "Do not put any code in this frame.\n(It is a separator no-op. You can make a copy of this frame to create a new Macro frame)"
        n95 = call <vilib>:"Add State(s) to Queue__JKI_lib_State_Machine.vi"("State(s) in Front (\"\")"="UI: Cursor Set >> Busy\nFile: Load\nGraph: Initialize Graphs" ("State(s) in Front (\"\")"), "State(s) in (\"\")"="Process Queue", "State(s) at Back (\"\")"="Graph: Update Graphs\nUI: Cursor Set >> Idle" ("State(s) in Front (\"\")")) -> ("States Out"=w249:string)  [unwired: 12 in]
        "Processed States" <- w249
        n96 = call <vilib>:"Add State(s) to Queue__JKI_lib_State_Machine.vi"("State(s) in Front (\"\")"=w249, "State(s) in (\"\")"=w256) -> ("States Out"=w255:string)  [unwired: 13 in]
      }
      frame "---------- Graph ----------" {
        # "Do not put any code in this frame.\n(It is a separator no-op. You can make a copy of this frame to create a new Macro frame)"
        n97 = call <vilib>:"Add State(s) to Queue__JKI_lib_State_Machine.vi"("State(s) in (\"\")"=w260) -> ("States Out"=w259:string)  [unwired: 14 in]
      }
      frame "Graph: Controls" {
        # "Do not put any code in this frame.\n(It is a separator no-op. You can make a copy of this frame to create a new Macro frame)"
        n98 = call <vilib>:"Add State(s) to Queue__JKI_lib_State_Machine.vi"("State(s) in (\"\")"=w264) -> ("States Out"=w263:string)  [unwired: 14 in]
      }
      frame "Graph: Initialize References 1" {
        # "Do not put any code in this frame.\n(It is a separator no-op. You can make a copy of this frame to create a new Data frame)"
        n99 = control-ref of="XY Graph: Unprocessed"() -> (w275:refnum<vi>)
        n100 = control-ref of="Data Intensity"() -> (w270:refnum<vi>)
        n101 = control-ref of="XY Graph: Processed"() -> (w269:refnum<vi>)
        n102 = call <userlib>:"Write Intensity Graph ref.vi"("error in (no error)"=w268, "Intensity Graph"=w270) -> ("error out"=w276:errorcluster, "graph_utilities out"=w274:refnum<class "graph_utilities.lvclass">)  [unwired: 8 in]
        n103 = call <userlib>:"Write Intensity Graph ref.vi"("error in (no error)"=w268, "Intensity Graph"=w270) -> ("error out"=w271:errorcluster, "graph_utilities out"=w266:refnum<class "graph_utilities.lvclass">)  [unwired: 8 in]
        n104 = call <userlib>:"Write XY Graph ref.vi"("error in (no error)"=w276, "XY Graph"=w275, "graph_utilities in"=w274) -> ("error out"=w272:errorcluster, "graph_utilities out"=w273:refnum<class "graph_utilities.lvclass">)  [unwired: 7 in]
        n105 = call <userlib>:"Write XY Graph ref.vi"("error in (no error)"=w271, "XY Graph"=w269, "graph_utilities in"=w266) -> ("error out"=w267:errorcluster, "graph_utilities out"=w265:refnum<class "graph_utilities.lvclass">)  [unwired: 7 in]
        n106 = Bundle By Name(cluster=w279, "Graph.Data: Unprocessed"=w273, "Graph.Data: Processed"=w265) -> (w278:T5)
        n107 = Merge Errors(w272, w267) -> (w277:errorcluster)
        n108 = call <vilib>:"Add State(s) to Queue__JKI_lib_State_Machine.vi"("State(s) in (\"\")"=w281) -> ("States Out"=w280:string)  [unwired: 14 in]
      }
      frame "Graph: Initialize References 2" {
        # "Do not put any code in this frame.\n(It is a separator no-op. You can make a copy of this frame to create a new Data frame)"
        n109 = control-ref of="Data Vertical"() -> (w301:refnum<vi>)
        n110 = control-ref of="Data Horizontal"() -> (w295:refnum<vi>)
        n111 = control-ref of="Diff Vertical"() -> (w300:refnum<vi>)
        n112 = control-ref of="Diff Horizontal"() -> (w298:refnum<vi>)
        n113 = control-ref of="Data Intensity"() -> (w283:refnum<vi>)
        n114 = control-ref of="Diff Intensity"() -> (w293:refnum<vi>)
        n115 = call <userlib>:"Write Intensity Graph ref.vi"("error in (no error)"=w282, "Intensity Graph (Control)"=w283, "Intensity Graph"=w283) -> ("error out"=w294:errorcluster, "graph_utilities out"=w296:refnum<class "graph_utilities.lvclass">)  [unwired: 7 in]
        n116 = call <userlib>:"Write Intensity Graph ref.vi"("error in (no error)"=w282, "Intensity Graph (Control)"=w283, "Intensity Graph"=w293) -> ("error out"=w297:errorcluster, "graph_utilities out"=w299:refnum<class "graph_utilities.lvclass">)  [unwired: 7 in]
        n117 = call <userlib>:"Write XY Graph ref.vi"("error in (no error)"=w294, "XY Graph"=w295, "graph_utilities in"=w296) -> ("error out"=w291:errorcluster, "graph_utilities out"=w286:refnum<class "graph_utilities.lvclass">)  [unwired: 7 in]
        n118 = call <userlib>:"Write XY Graph ref.vi"("error in (no error)"=w297, "XY Graph"=w298, "graph_utilities in"=w299) -> ("error out"=w292:errorcluster, "graph_utilities out"=w284:refnum<class "graph_utilities.lvclass">)  [unwired: 7 in]
        n119 = call <userlib>:"Write XY Graph ref.vi"("error in (no error)"=w291, "XY Graph"=w301, "graph_utilities in"=w296) -> ("error out"=w290:errorcluster, "graph_utilities out"=w287:refnum<class "graph_utilities.lvclass">)  [unwired: 7 in]
        n120 = call <userlib>:"Write XY Graph ref.vi"("error in (no error)"=w292, "XY Graph"=w300, "graph_utilities in"=w299) -> ("error out"=w289:errorcluster, "graph_utilities out"=w285:refnum<class "graph_utilities.lvclass">)  [unwired: 7 in]
        n121 = Bundle By Name(cluster=w303, "Graph.Data: Intensity/Vertical"=w287, "Graph.Data: Intensity/Horizontal"=w286, "Graph.Differential: Intensity/Vertical"=w285, "Graph.Differential: Intensity/Horizontal"=w284) -> (w302:T5)
        n122 = Merge Errors(w290, w289) -> (w288:errorcluster)
        n123 = call <vilib>:"Add State(s) to Queue__JKI_lib_State_Machine.vi"("State(s) in (\"\")"=w305) -> ("States Out"=w304:string)  [unwired: 14 in]
      }
      frame "Graph: Initialize Graphs" {
        # "Do not put any code in this frame.\n(It is a separator no-op. You can make a copy of this frame to create a new Macro frame)"
        n124 = Unbundle By Name(w310) -> ("Graph.Data: Unprocessed"=w313:refnum<class "graph_utilities.lvclass">, "XY Data (unprocessed)"=w308:cluster{"Intensity Data":dbl[], "Array":dbl[]}[], "Parameter"=w307:dbl[])
        n125 = call-poly <userlib>:"Set XY Graph Value.vi"("error in (no error)"=w309, "Value"=w308, "graph_utilities in"=w313) -> ("error out"=w312:errorcluster, "graph_utilities out"=w311:refnum<class "graph_utilities.lvclass">)  [unwired: 7 in]
        n126 = call <userlib>:"XY Graph to Intensity Graph.vi"("error in (no error)"=w312, "Y Scale"=w307, "graph_utilities in"=w311) -> ("error out"=w306:errorcluster)  [unwired: 7 in, 1 out]
        n127 = call <vilib>:"Add State(s) to Queue__JKI_lib_State_Machine.vi"("State(s) in (\"\")"=w315) -> ("States Out"=w314:string)  [unwired: 14 in]
      }
      frame "Graph: Update Graphs" {
        # "Do not put any code in this frame.\n(It is a separator no-op. You can make a copy of this frame to create a new UI frame)"
        n128 = Unbundle By Name(w323) -> ("Graph.Data: Processed"=w322:refnum<class "graph_utilities.lvclass">, "XY Data (processed 1)"=w321:cluster{"Intensity Data":dbl[], "Array":dbl[]}[], "Parameter"=w318:dbl[])
        n129 = call-poly <userlib>:"Set XY Graph Value.vi"("error in (no error)"=w320, "Value"=w321, "graph_utilities in"=w322) -> ("error out"=w317:errorcluster, "graph_utilities out"=w319:refnum<class "graph_utilities.lvclass">)  [unwired: 7 in]
        n130 = call <userlib>:"XY Graph to Intensity Graph.vi"("error in (no error)"=w317, "Y Scale"=w318, "graph_utilities in"=w319) -> ("error out"=w316:errorcluster)  [unwired: 7 in, 1 out]
        n131 = call <vilib>:"Add State(s) to Queue__JKI_lib_State_Machine.vi"("State(s) in (\"\")"=w325) -> ("States Out"=w324:string)  [unwired: 14 in]
      }
      frame "Graph: Clear" {
        w326 = cluster{dbl[], dbl[]}[] [] ("Value")
        w329 = dbl[][] [] ("Value")
        # "Do not put any code in this frame.\n(It is a separator no-op. You can make a copy of this frame to create a new Macro frame)"
        n132 = Unbundle By Name(w346) -> ("Graph.Data: Unprocessed"=w330:refnum<class "graph_utilities.lvclass">, "Graph.Data: Processed"=w345:refnum<class "graph_utilities.lvclass">, "Graph.Data: Intensity/Vertical"=w339:refnum<class "graph_utilities.lvclass">, "Graph.Data: Intensity/Horizontal"=w338:refnum<class "graph_utilities.lvclass">, "Graph.Differential: Intensity/Vertical"=w337:refnum<class "graph_utilities.lvclass">, "Graph.Differential: Intensity/Horizontal"=w336:refnum<class "graph_utilities.lvclass">)
        n133 = call <userlib>:"Set Intensity Graph Value.vi"("Value"=w329, "graph_utilities in"=w330) -> ("error out"=w327:errorcluster, "graph_utilities out"=w328:refnum<class "graph_utilities.lvclass">)  [unwired: 8 in]
        n134 = call <userlib>:"Set Intensity Graph Value.vi"("Value"=w329, "graph_utilities in"=w345) -> ("error out"=w335:errorcluster, "graph_utilities out"=w344:refnum<class "graph_utilities.lvclass">)  [unwired: 8 in]
        n135 = call <userlib>:"Set Intensity Graph Value.vi"("Value"=w329, "graph_utilities in"=w338) -> ("error out"=w333:errorcluster, "graph_utilities out"=w342:refnum<class "graph_utilities.lvclass">)  [unwired: 8 in]
        n136 = call <userlib>:"Set Intensity Graph Value.vi"("Value"=w329, "graph_utilities in"=w339) -> ("error out"=w334:errorcluster, "graph_utilities out"=w343:refnum<class "graph_utilities.lvclass">)  [unwired: 8 in]
        n137 = call <userlib>:"Set Intensity Graph Value.vi"("Value"=w329, "graph_utilities in"=w337) -> ("error out"=w332:errorcluster, "graph_utilities out"=w341:refnum<class "graph_utilities.lvclass">)  [unwired: 8 in]
        n138 = call <userlib>:"Set Intensity Graph Value.vi"("Value"=w329, "graph_utilities in"=w336) -> ("error out"=w331:errorcluster, "graph_utilities out"=w340:refnum<class "graph_utilities.lvclass">)  [unwired: 8 in]
        n139 = call-poly <userlib>:"Set XY Graph Value.vi"("error in (no error)"=w327, "Value"=w326, "graph_utilities in"=w328) -> ()  [unwired: 7 in, 2 out]
        n140 = call-poly <userlib>:"Set XY Graph Value.vi"("error in (no error)"=w335, "Value"=w326, "graph_utilities in"=w344) -> ()  [unwired: 7 in, 2 out]
        n141 = call-poly <userlib>:"Set XY Graph Value.vi"("error in (no error)"=w333, "Value"=w326, "graph_utilities in"=w342) -> ()  [unwired: 7 in, 2 out]
        n142 = call-poly <userlib>:"Set XY Graph Value.vi"("error in (no error)"=w334, "Value"=w326, "graph_utilities in"=w343) -> ()  [unwired: 7 in, 2 out]
        n143 = call-poly <userlib>:"Set XY Graph Value.vi"("error in (no error)"=w332, "Value"=w326, "graph_utilities in"=w341) -> ()  [unwired: 7 in, 2 out]
        n144 = call-poly <userlib>:"Set XY Graph Value.vi"("error in (no error)"=w331, "Value"=w326, "graph_utilities in"=w340) -> ()  [unwired: 7 in, 2 out]
        n145 = local write "XY Graph: Antisymmetric"(w326) -> ()
        n146 = local write "XY Graph: Symmetric"(w326) -> ()
        n147 = call <vilib>:"Add State(s) to Queue__JKI_lib_State_Machine.vi"("State(s) in (\"\")"=w349) -> ("States Out"=w348:string)  [unwired: 14 in]
      }
      frame "Graph: Linecut" {
        # "Do not put any code in this frame.\n(It is a separator no-op. You can make a copy of this frame to create a new Macro frame)"
        n148 = Unbundle By Name(w363) -> ("Graph.Data: Intensity/Vertical"=w362:refnum<class "graph_utilities.lvclass">, "Graph.Data: Intensity/Horizontal"=w361:refnum<class "graph_utilities.lvclass">, "Graph.Differential: Intensity/Vertical"=w360:refnum<class "graph_utilities.lvclass">, "Graph.Differential: Intensity/Horizontal"=w359:refnum<class "graph_utilities.lvclass">)
        n149 = call <userlib>:"Intensity Graph Linecut (Vertical).vi"("error in (no error)"=w356, "width (vertical)"="width (vertical)", "graph_utilities in"=w362) -> ("error out"=w357:errorcluster)  [unwired: 7 in, 1 out]
        n150 = call <userlib>:"Intensity Graph Linecut (Horizontal).vi"("error in (no error)"=w357, "width (horizontal)"="width (horizontal)", "graph_utilities in"=w361) -> ("error out"=w358:errorcluster)  [unwired: 7 in, 1 out]
        n151 = call <userlib>:"Intensity Graph Linecut (Vertical).vi"("error in (no error)"=w358, "width (vertical)"="width (vertical) 2", "graph_utilities in"=w360) -> ("error out"=w355:errorcluster)  [unwired: 7 in, 1 out]
        n152 = call <userlib>:"Intensity Graph Linecut (Horizontal).vi"("error in (no error)"=w355, "width (horizontal)"="width (horizontal) 2", "graph_utilities in"=w359) -> ("error out"=w354:errorcluster)  [unwired: 7 in, 1 out]
        n153 = call <vilib>:"Add State(s) to Queue__JKI_lib_State_Machine.vi"("State(s) in (\"\")"=w365) -> ("States Out"=w364:string)  [unwired: 14 in]
      }
      frame "---------- File ----------" {
        # "Do not put any code in this frame.\n(It is a separator no-op. You can make a copy of this frame to create a new Macro frame)"
        n154 = call <vilib>:"Add State(s) to Queue__JKI_lib_State_Machine.vi"("State(s) in (\"\")"=w369) -> ("States Out"=w368:string)  [unwired: 14 in]
      }
      frame "File: Load" {
        # "Add code here for loading your data from disk"
        # "File: Load\n(Add code here for loading your data)"
        n155 = disable-structure shown="Enabled" {
          disable-tunnel: [w382 w384] -> w371
          disable-tunnel: cluster{"Intensity Data":dbl[], "Array":dbl[]}[] [{"Intensity Data"=[0.0, 0.004, 0.008, 0.012, 0.016, 0.02, 0.024, 0.028, 0.032, 0.036000000000000004, 0.04, 0.044, 0.048, 0.052000000000000005, 0.056, 0.06, 0.064, 0.068, 0.07200000000000001, 0.076, 0.08, 0.084, 0.088, 0.092, 0.096, 0.1, 0.10400000000000001, 0.108, 0.112, 0.116, 0.12, 0.124, 0.128, 0.132, 0.136, 0.14, 0.14400000000000002, 0.148, 0.152, 0.156, 0.16, 0.164, 0.168, 0.17200000000000001, 0.176, 0.18, 0.184, 0.188, 0.192, 0.196, 0.2, 0.20400000000000001, 0.20800000000000002, 0.212, 0.216, 0.22, 0.224, 0.228, 0.232, 0.23600000000000002, 0.24, 0.244, 0.248, 0.252, 0.256, 0.26, 0.264, 0.268, 0.272, 0.276, 0.28, 0.28400000000000003, 0.28800000000000003, 0.292, 0.296, 0.3, 0.304, 0.308, 0.312, 0.316, 0.32, 0.324, 0.328, 0.332, 0.336, 0.34, 0.34400000000000003, 0.34800000000000003, 0.352, 0.356, 0.36, 0.364, 0.368, 0.372, 0.376, 0.38, 0.384, 0.388, 0.392, 0.396, 0.4, 0.404, 0.40800000000000003, 0.41200000000000003, 0.41600000000000004, 0.42, 0.424, 0.428, 0.432, 0.436, 0.44, 0.444, 0.448, 0.452, 0.456, 0.46, 0.464, 0.468, 0.47200000000000003, 0.47600000000000003, 0.48, 0.484, 0.488, 0.492, 0.496, 0.5, 0.504, 0.508, 0.512, 0.516, 0.52, 0.524, 0.528, 0.532, 0.536, 0.54, 0.544, 0.548, 0.552, 0.556, 0.56, 0.5640000000000001, 0.5680000000000001, 0.5720000000000001, 0.5760000000000001, 0.58, 0.584, 0.588, 0.592, 0.596, 0.6, 0.604, 0.608, 0.612, 0.616, 0.62, 0.624, 0.628, 0.632, 0.636, 0.64, 0.644, 0.648, 0.652, 0.656, 0.66, 0.664, 0.668, 0.672, 0.676, 0.68, 0.684, 0.6880000000000001, 0.6920000000000001, 0.6960000000000001, 0.7000000000000001, 0.704, 0.708, 0.712, 0.716, 0.72, 0.724, 0.728, 0.732, 0.736, 0.74, 0.744, 0.748, 0.752, 0.756, 0.76, 0.764, 0.768, 0.772, 0.776, 0.78, 0.784, 0.788, 0.792, 0.796, 0.8, 0.804, 0.808, 0.812, 0.8160000000000001, 0.8200000000000001, 0.8240000000000001, 0.8280000000000001, 0.8320000000000001, 0.836, 0.84, 0.844, 0.848, 0.852, 0.856, 0.86, 0.864, 0.868, 0.872, 0.876, 0.88], "Array"=[1.68063e-07, 1.37198e-07, 8.79687e-08, 1.06463e-07, 1.07999e-07, 1.50443e-07, 1.6136e-07, 1.60216e-07, 1.51628e-07, 1.62347e-07, 2.24052e-07, 2.12498e-07, 1.69888e-07, 2.07771e-07, 2.10504e-07, 1.16164e-07, 1.03648e-07, 1.88353e-07, 2.52956e-07, 1.81322e-07, 1.3598e-07, 1.93502e-07, 3.06623e-07, 1.81397e-07, 1.56136e-07, 7.65771e-08, 1.0323e-07, 2.25052e-07, 2.18994e-07, 1.48687e-07, 1.23465e-07, 1.94812e-07, 8.89733e-08, 1.01215e-07, 1.91375e-07, 1.83998e-07, 1.70281e-07, 2.66741e-07, 1.84557e-07, 1.35922e-07, 1.53284e-07, 1.28241e-07, 1.84801e-07, 1.04068e-07, 8.03285e-08, 1.04402e-07, 8.12206e-08, 5.15301e-08, 2.02427e-07, 1.78907e-07, 1.0348e-07, 8.96397e-08, 1.49064e-07, 2.10614e-07, 1.94321e-07, 1.23458e-07, 2.49381e-08, 1.85551e-07, 1.98644e-07, 2.30779e-07, 3.77495e-07, 6.72036e-07, 1.17947e-06, 1.75588e-06, 2.53801e-06, 3.50995e-06, 4.10398e-06, 4.4421e-06, 4.54957e-06, 4.46684e-06, 4.29614e-06, 4.03689e-06, 3.7785e-06, 3.52652e-06, 3.3015e-06, 3.0176e-06, 2.73351e-06, 2.48081e-06, 2.28944e-06, 2.06704e-06, 1.80961e-06, 1.62787e-06, 1.44499e-06, 1.27341e-06, 1.12003e-06, 1.00442e-06, 8.63595e-07, 7.29893e-07, 6.0347e-07, 5.41881e-07, 4.90755e-07, 4.14075e-07, 3.64346e-07, 3.41478e-07, 3.11551e-07, 2.93279e-07, 3.09014e-07, 3.23829e-07, 3.14767e-07, 3.13298e-07, 3.2943e-07, 3.73559e-07, 3.85052e-07, 4.12776e-07, 4.52513e-07, 4.63779e-07, 5.00565e-07, 5.25226e-07, 5.28226e-07, 5.09122e-07, 4.69838e-07, 4.77525e-07, 4.87608e-07, 4.64681e-07, 4.29366e-07, 4.10075e-07, 3.911e-07, 3.53091e-07, 3.11529e-07, 2.80052e-07, 2.48962e-07, 2.2069e-07, 2.00389e-07, 1.80056e-07, 1.71025e-07, 1.52747e-07, 1.20455e-07, 1.10317e-07, 1.22804e-07, 1.19285e-07, 1.05556e-07, 1.00514e-07, 1.16004e-07, 1.33715e-07, 1.48638e-07, 1.67858e-07, 1.60768e-07, 1.72191e-07, 1.90163e-07, 2.12957e-07, 2.27031e-07, 2.42395e-07, 2.5957e-07, 2.75457e-07, 2.81378e-07, 2.87991e-07, 2.8598e-07, 2.99029e-07, 3.10983e-07, 2.98582e-07, 2.92597e-07, 2.96466e-07, 2.75316e-07, 2.60924e-07, 2.73094e-07, 2.76228e-07, 2.69051e-07, 2.49348e-07, 2.40239e-07, 2.38694e-07, 2.46997e-07, 2.3754e-07, 2.31936e-07, 2.37921e-07, 2.4129e-07, 2.36577e-07, 2.27175e-07, 2.23179e-07, 2.32753e-07, 2.22017e-07, 2.21659e-07, 2.35338e-07, 2.45551e-07, 2.48375e-07, 2.61624e-07, 2.68417e-07, 2.63606e-07, 2.83272e-07, 2.96328e-07, 2.89196e-07, 2.96568e-07, 3.03707e-07, 3.06523e-07, 3.1915e-07, 3.12655e-07, 2.95357e-07, 2.95008e-07, 2.98448e-07, 3.09012e-07, 3.01923e-07, 2.96206e-07, 3.10244e-07, 3.04155e-07, 2.92192e-07, 2.85057e-07, 2.82269e-07, 2.90168e-07, 2.75276e-07, 2.42554e-07, 2.36848e-07, 2.39448e-07, 2.14838e-07, 2.06682e-07, 2.0462e-07, 1.85893e-07, 1.77192e-07, 1.71389e-07, 1.56772e-07, 1.51419e-07, 1.47796e-07, 1.53989e-07, 1.38128e-07, 1.40478e-07, 1.52301e-07, 1.42379e-07, 1.31716e-07, 1.3604e-07, 1.51662e-07, 1.43388e-07, 1.35586e-07, 1.45146e-07]}, ...(73 in all)] ("Vertical") -> [_ w384]
          disable-tunnel: dbl[] [-9.0, -8.75, -8.5, -8.25, -8.0, -7.75, -7.5, -7.25, -7.0, -6.75, -6.5, -6.25, -6.0, -5.75, -5.5, -5.25, -5.0, -4.75, -4.5, -4.25, -4.0, -3.75, -3.5, -3.25, -3.0, -2.75, -2.5, -2.25, -2.0, -1.75, -1.5, -1.25, -1.0, -0.75, -0.5, -0.25, 0.0, 0.25, 0.5, 0.75, 1.0, 1.25, 1.5, 1.75, 2.0, 2.25, 2.5, 2.75, 3.0, 3.25, 3.5, 3.75, 4.0, 4.25, 4.5, 4.75, 5.0, 5.25, 5.5, 5.75, 6.0, 6.25, 6.5, 6.75, 7.0, 7.25, 7.5, 7.75, 8.0, 8.25, 8.5, 8.75, 9.0] ("X") -> [_ w383]
          disable-tunnel: [w379 w383] -> w372
          frame Disabled {
            n156 = call <userlib>:"LV to ITX  Retrieve.vi"() -> ("A vs B"=w382:cluster{dbl[], dbl[]}[], "N"=w381:cluster{"N1":dbl, "N2":dbl, "N3":dbl, "N4":dbl})  [unwired: 11 in, 3 out]
            n157 = Unbundle By Name(w381) -> ("N1"=w380:dbl)
            n158 = Build Array(w380) -> (w379:dbl[])
          }
          frame Enabled {
          }
        }
        n159 = Bundle By Name(cluster=w373, "XY Data (unprocessed)"=w371, "XY Data (processed 1)"=w371, "XY Data (processed 2)"=w371, "Parameter"=w372) -> (w376:T5)
        n160 = call <vilib>:"Add State(s) to Queue__JKI_lib_State_Machine.vi"("State(s) in (\"\")"=w378) -> ("States Out"=w377:string)  [unwired: 14 in]
      }
      frame "---------- XY ----------" {
        # "Template Separator\n(You can make a copy of, or modify, this frame)"
        n161 = Unbundle By Name(w389) -> ("XY Data (processed 1)"=w390:cluster{"Intensity Data":dbl[], "Array":dbl[]}[])
        n162 = call-poly <userlib>:"Add.vi"("error in (no error)"=w386, "XY-data"=w390) -> ("error out"=w385:errorcluster, "XY-data out"=w387:cluster{"X-array":dbl[], "Y-array":dbl[]}[])  [unwired: 8 in]
        n163 = Bundle By Name(cluster=w389, "XY Data (processed 1)"=w387) -> (w388:T5)
        n164 = call <vilib>:"Add State(s) to Queue__JKI_lib_State_Machine.vi"("State(s) in (\"\")"=w392) -> ("States Out"=w391:string)  [unwired: 14 in]
      }
      frame "XY: Add" {
        # "XY: Add\n(You can make a copy of, or modify, this frame)"
        n165 = Unbundle By Name(w399) -> ("XY Data (processed 1)"=w400:cluster{"Intensity Data":dbl[], "Array":dbl[]}[])
        n166 = call-poly <userlib>:"Add.vi"("error in (no error)"=w396, "y (0)"="y", "x (0)"="x", "XY-data"=w400) -> ("error out"=w395:errorcluster, "XY-data out"=w397:cluster{"X-array":dbl[], "Y-array":dbl[]}[])  [unwired: 6 in]
        n167 = Bundle By Name(cluster=w399, "XY Data (processed 1)"=w397) -> (w398:T5)
        n168 = call <vilib>:"Add State(s) to Queue__JKI_lib_State_Machine.vi"("State(s) in (\"\")"=w402) -> ("States Out"=w401:string)  [unwired: 14 in]
      }
      frame "XY: Subtract" {
        # "Template Separator\n(You can make a copy of, or modify, this frame)"
        n169 = Unbundle By Name(w409) -> ("XY Data (processed 1)"=w410:cluster{"Intensity Data":dbl[], "Array":dbl[]}[])
        n170 = local read "x"() -> (w403:dbl)
        n171 = local read "y"() -> (w404:dbl)
        n172 = call-poly <userlib>:"Subtract.vi"("error in (no error)"=w406, "y (0)"=w404, "x (0)"=w403, "XY-data"=w410) -> ("error out"=w405:errorcluster, "XY-data out"=w407:cluster{"X-array":dbl[], "Y-array":dbl[]}[])  [unwired: 6 in]
        n173 = Bundle By Name(cluster=w409, "XY Data (processed 1)"=w407) -> (w408:T5)
        n174 = call <vilib>:"Add State(s) to Queue__JKI_lib_State_Machine.vi"("State(s) in (\"\")"=w412) -> ("States Out"=w411:string)  [unwired: 14 in]
      }
      frame "XY: Multiply" {
        # "Template Separator\n(You can make a copy of, or modify, this frame)"
        n175 = Unbundle By Name(w419) -> ("XY Data (processed 1)"=w420:cluster{"Intensity Data":dbl[], "Array":dbl[]}[])
        n176 = local read "x"() -> (w414:dbl)
        n177 = local read "y"() -> (w413:dbl)
        n178 = call-poly <userlib>:"Multiply.vi"("error in (no error)"=w416, "y (1)"=w413, "x (1)"=w414, "XY-data"=w420) -> ("error out"=w415:errorcluster, "XY-data out"=w417:cluster{"X-array":dbl[], "Y-array":dbl[]}[])  [unwired: 6 in]
        n179 = Bundle By Name(cluster=w419, "XY Data (processed 1)"=w417) -> (w418:T5)
        n180 = call <vilib>:"Add State(s) to Queue__JKI_lib_State_Machine.vi"("State(s) in (\"\")"=w422) -> ("States Out"=w421:string)  [unwired: 14 in]
      }
      frame "XY: Square" {
        # "Template Separator\n(You can make a copy of, or modify, this frame)"
        n181 = Unbundle By Name(w427) -> ("XY Data (processed 1)"=w428:cluster{"Intensity Data":dbl[], "Array":dbl[]}[])
        n182 = call-poly <userlib>:"Square.vi"("error in (no error)"=w424, "XY-data"=w428) -> ("error out"=w423:errorcluster, "XY-data out"=w425:cluster{"X-array":dbl[], "Y-array":dbl[]}[])  [unwired: 8 in]
        n183 = Bundle By Name(cluster=w427, "XY Data (processed 1)"=w425) -> (w426:T5)
        n184 = call <vilib>:"Add State(s) to Queue__JKI_lib_State_Machine.vi"("State(s) in (\"\")"=w430) -> ("States Out"=w429:string)  [unwired: 14 in]
      }
      frame "XY: Divide" {
        # "Template Separator\n(You can make a copy of, or modify, this frame)"
        n185 = Unbundle By Name(w437) -> ("XY Data (processed 1)"=w438:cluster{"Intensity Data":dbl[], "Array":dbl[]}[])
        n186 = local read "x"() -> (w432:dbl)
        n187 = local read "y"() -> (w431:dbl)
        n188 = call-poly <userlib>:"Divide.vi"("error in (no error)"=w434, "y (1)"=w431, "x (1)"=w432, "XY-data"=w438) -> ("error out"=w433:errorcluster, "XY-data out"=w435:cluster{"X-array":dbl[], "Y-array":dbl[]}[])  [unwired: 6 in]
        n189 = Bundle By Name(cluster=w437, "XY Data (processed 1)"=w435) -> (w436:T5)
        n190 = call <vilib>:"Add State(s) to Queue__JKI_lib_State_Machine.vi"("State(s) in (\"\")"=w440) -> ("States Out"=w439:string)  [unwired: 14 in]
      }
      frame "XY: Sort" {
        # "Template Separator\n(You can make a copy of, or modify, this frame)"
        n191 = Unbundle By Name(w445) -> ("XY Data (processed 1)"=w446:cluster{"Intensity Data":dbl[], "Array":dbl[]}[])
        n192 = call-poly <userlib>:"Sort.vi"("error in (no error)"=w442, "XY-data"=w446) -> ("error out"=w441:errorcluster, "Sorted XY-data out"=w443:cluster{"X-array":dbl[], "Y-array":dbl[]}[])  [unwired: 8 in]
        n193 = Bundle By Name(cluster=w445, "XY Data (processed 1)"=w443) -> (w444:T5)
        n194 = call <vilib>:"Add State(s) to Queue__JKI_lib_State_Machine.vi"("State(s) in (\"\")"=w448) -> ("States Out"=w447:string)  [unwired: 14 in]
      }
      frame "XY: Swap" {
        # "Template Separator\n(You can make a copy of, or modify, this frame)"
        n195 = Unbundle By Name(w453) -> ("XY Data (processed 1)"=w454:cluster{"Intensity Data":dbl[], "Array":dbl[]}[])
        n196 = call-poly <userlib>:"Swap X and Y.vi"("error in (no error)"=w450, "XY-data"=w454) -> ("error out"=w449:errorcluster, "XY-data out"=w451:cluster{"X-array":dbl[], "Y-array":dbl[]}[])  [unwired: 8 in]
        n197 = Bundle By Name(cluster=w453, "XY Data (processed 1)"=w451) -> (w452:T5)
        n198 = call <vilib>:"Add State(s) to Queue__JKI_lib_State_Machine.vi"("State(s) in (\"\")"=w456) -> ("States Out"=w455:string)  [unwired: 14 in]
      }
      frame "XY: Reverse" {
        # "Template Separator\n(You can make a copy of, or modify, this frame)"
        n199 = Unbundle By Name(w461) -> ("XY Data (processed 1)"=w462:cluster{"Intensity Data":dbl[], "Array":dbl[]}[])
        n200 = call-poly <userlib>:"Reverse.vi"("error in (no error)"=w458, "XY-data"=w462) -> ("error out"=w457:errorcluster, "Reversed XY-data out"=w459:cluster{"X-array":dbl[], "Y-array":dbl[]}[])  [unwired: 8 in]
        n201 = Bundle By Name(cluster=w461, "XY Data (processed 1)"=w459) -> (w460:T5)
        n202 = call <vilib>:"Add State(s) to Queue__JKI_lib_State_Machine.vi"("State(s) in (\"\")"=w464) -> ("States Out"=w463:string)  [unwired: 14 in]
      }
      frame "XY: Subset" {
        # "Template Separator\n(You can make a copy of, or modify, this frame)"
        n203 = Unbundle By Name(w471) -> ("XY Data (processed 1)"=w472:cluster{"Intensity Data":dbl[], "Array":dbl[]}[])
        n204 = call-poly <userlib>:"Subset.vi"("error in (no error)"=w468, "Subset Method"="Method", "Subset Slider"="Subset Slider", "XY-data"=w472) -> ("error out"=w467:errorcluster, "Subset XY-data out"=w469:cluster{"X-array":dbl[], "Y-array":dbl[]}[])  [unwired: 6 in]
        n205 = Bundle By Name(cluster=w471, "XY Data (processed 1)"=w469) -> (w470:T5)
        n206 = call <vilib>:"Add State(s) to Queue__JKI_lib_State_Machine.vi"("State(s) in (\"\")"=w474) -> ("States Out"=w473:string)  [unwired: 14 in]
      }
      frame "XY: Derivative" {
        # "Template Separator\n(You can make a copy of, or modify, this frame)"
        n207 = Unbundle By Name(w482) -> ("XY Data (processed 1)"=w483:cluster{"Intensity Data":dbl[], "Array":dbl[]}[])
        n208 = call-poly <userlib>:"Derivative.vi"("Interval Units"="Interval Units", "error in (no error)"=w480, "Type"="Type", "Interval"="Interval", "XY-data"=w483) -> ("error out"=w479:errorcluster, "Differential out"=w475:cluster{"X-array":dbl[], "Y-array":dbl[]}[])  [unwired: 4 in, 1 out]
        n209 = Bundle By Name(cluster=w482, "XY Data (processed 1)"=w475) -> (w481:T5)
        n210 = call <vilib>:"Add State(s) to Queue__JKI_lib_State_Machine.vi"("State(s) in (\"\")"=w485) -> ("States Out"=w484:string)  [unwired: 14 in]
      }
      frame "XY: Interpolate" {
        # "Template Separator\n(You can make a copy of, or modify, this frame)"
        n211 = Unbundle By Name(w491) -> ("XY Data (processed 1)"=w492:cluster{"Intensity Data":dbl[], "Array":dbl[]}[])
        n212 = call-poly <userlib>:"Interpolate.vi"("error in (no error)"=w488, "Configure"="Configure", "XY-data"=w492) -> ("error out"=w487:errorcluster, "Interpolated XY-data out"=w489:cluster{"X-array":dbl[], "Y-array":dbl[]}[])  [unwired: 7 in]
        n213 = Bundle By Name(cluster=w491, "XY Data (processed 1)"=w489) -> (w490:T5)
        n214 = call <vilib>:"Add State(s) to Queue__JKI_lib_State_Machine.vi"("State(s) in (\"\")"=w494) -> ("States Out"=w493:string)  [unwired: 14 in]
      }
      frame "XY: FFT Spectrum" {
        # "Template Separator\n(You can make a copy of, or modify, this frame)"
        n215 = Unbundle By Name(w499) -> ("XY Data (processed 1)"=w500:cluster{"Intensity Data":dbl[], "Array":dbl[]}[])
        n216 = call-poly <userlib>:"FFT Spectrum.vi"("error in (no error)"=w496, "XY-data"=w500) -> ("error out"=w495:errorcluster, "XY-data out"=w497:cluster{"X-array":dbl[], "Y-array":dbl[]}[])  [unwired: 6 in, 2 out]
        n217 = Bundle By Name(cluster=w499, "XY Data (processed 1)"=w497) -> (w498:T5)
        n218 = call <vilib>:"Add State(s) to Queue__JKI_lib_State_Machine.vi"("State(s) in (\"\")"=w502) -> ("States Out"=w501:string)  [unwired: 14 in]
      }
      frame "XY: FFT Power Spectrum" {
        # "Template Separator\n(You can make a copy of, or modify, this frame)"
        n219 = Unbundle By Name(w507) -> ("XY Data (processed 1)"=w508:cluster{"Intensity Data":dbl[], "Array":dbl[]}[])
        n220 = call-poly <userlib>:"FFT Power Spectrum.vi"("error in (no error)"=w505, "XY-data"=w508) -> ("error out"=w504:errorcluster, "XY-data out"=w503:cluster{"X-array":dbl[], "Y-array":dbl[]}[])  [unwired: 7 in, 1 out]
        n221 = Bundle By Name(cluster=w507, "XY Data (processed 1)"=w503) -> (w506:T5)
        n222 = call <vilib>:"Add State(s) to Queue__JKI_lib_State_Machine.vi"("State(s) in (\"\")"=w510) -> ("States Out"=w509:string)  [unwired: 14 in]
      }
      frame "XY: Resample" {
        # "Template Separator\n(You can make a copy of, or modify, this frame)"
        n223 = Unbundle By Name(w515) -> ("XY Data (processed 1)"=w516:cluster{"Intensity Data":dbl[], "Array":dbl[]}[])
        n224 = call-poly <userlib>:"Resample.vi"("error in (no error)"=w512, "XY-data"=w516) -> ("error out"=w511:errorcluster, "Resampled XY-data out"=w513:cluster{"X-array":dbl[], "Y-array":dbl[]}[])  [unwired: 8 in]
        n225 = Bundle By Name(cluster=w515, "XY Data (processed 1)"=w513) -> (w514:T5)
        n226 = call <vilib>:"Add State(s) to Queue__JKI_lib_State_Machine.vi"("State(s) in (\"\")"=w518) -> ("States Out"=w517:string)  [unwired: 14 in]
      }
      frame "XY: Average" {
        # "Template Separator\n(You can make a copy of, or modify, this frame)"
        n227 = Unbundle By Name(w523) -> ("XY Data (processed 1)"=w524:cluster{"Intensity Data":dbl[], "Array":dbl[]}[])
        n228 = call <userlib>:"Average.vi"("error in (no error)"=w520, "XY-data"=w524) -> ("error out"=w519:errorcluster, "XY-data out"=w521:cluster{"X-array":dbl[], "Y-array":dbl[]}[])  [unwired: 7 in, 1 out]
        n229 = Bundle By Name(cluster=w523, "XY Data (processed 1)"=w521) -> (w522:T5)
        n230 = call <vilib>:"Add State(s) to Queue__JKI_lib_State_Machine.vi"("State(s) in (\"\")"=w526) -> ("States Out"=w525:string)  [unwired: 14 in]
      }
      frame "XY: Symmeterize" {
        # "Template Separator\n(You can make a copy of, or modify, this frame)"
        n231 = Unbundle By Name(w533) -> ("XY Data (processed 1)"=w534:cluster{"Intensity Data":dbl[], "Array":dbl[]}[])
        n232 = call-poly <userlib>:"Symmetrize.vi"("error in (no error)"=w530, "XY-data"=w534) -> ("error out"=w529:errorcluster, "Antisymmetric"=→"XY Graph: Antisymmetric":cluster{"X-array":dbl[], dbl[]}[], "Symmetric"=→"XY Graph: Symmetric":cluster{"X-array":dbl[], dbl[]}[], "XY-data out"=w531:cluster{"X-array":dbl[], "Y-array":dbl[]}[])  [unwired: 6 in]
        n233 = Bundle By Name(cluster=w533, "XY Data (processed 1)"=w531) -> (w532:T5)
        n234 = call <vilib>:"Add State(s) to Queue__JKI_lib_State_Machine.vi"("State(s) in (\"\")"=w536) -> ("States Out"=w535:string)  [unwired: 14 in]
      }
    }
  }
